vi "UHR-Fleezers Control (fpga) - 10.8a.vi"() -> ()   [LabVIEW 2014]
doc: "UHR-Fleezers Instrument Control Code (fpga)"
uses:
  <vilib>/eio/EIONode/EIONode.xnode
  <vilib>/eio/EIOMethodNode/EIOMethodNode.xnode
  <vilib>/rvi/DataTransferAndStorage/Container/XNode/niFpgaContainer.xnode
  <vilib>/Platform/TimedLoop/XDataNode/XDataNode.xnode
  <vilib>/Platform/TimedLoop/XDataNode/nitl_modes.ctl
  <vilib>/Platform/TimedLoop/XDataNode/XDNodeRunTimeDep.lvlib
  <vilib>/Platform/TimedLoop/XDataNode/wakeup.ctl
  <vilib>/Platform/TimedLoop/XDataNode/timing_clust.ctl
  <vilib>/addons/control/pid/fpga.llb/XNode/niFpgaPID.xnode
  <vilib>/rvi/eio/common/nirviEmuTemplateMethod_errors.vi
  <vilib>/rvi/interface/RandomDataEmulation/nirviRandomDataFpgaReadWriteTemplate.vi
panel:
  in  "Connector0/AO6":i16
  in  "Tab Control":T1(tab)=enum."Force FB"
  in  "Trap Pos to FIFO":bool
  in  "AI1 Sets to FIFO":T2={"Set 1"=TRUE, "Set 2"=TRUE, "Set 3"=FALSE}
  in  "N of AI1 Int Acq Sets":i16=2 min=1 max=3 step=1
  out "AI Late Counter":u16
  in  "ai count":u32=400
  out "AI late?":bool
  in  "+ phase":bool
  in  "Phase count adjustment":i16
  out "Relative phase":i16
  in  "AI to FIFO":bool
  out "BD1 Frequency Out 1":u64
  out "BD1 Frequency Out 2":u64
  out "Trap Pos FIFO Timeout":u16
  out "Trap AI FIFO Timeout":u16
  in  "Trap FIFO Set Timeout":i32
  in  "Tab Control 2":T3(tab)
  out "Wiggling 2":bool
  in  "Abort wiggle 2":bool
  in  "Wiggle amp 2":u64
  in  "Wiggle freq 2 (Hz)":fxp<+/-,16,16>
  in  "Wiggle trap 2":bool
  out "Wiggling 1":bool
  in  "Abort wiggle 1":bool
  in  "Wiggle trap 1":bool
  in  "Wiggle amp 1":u64
  in  "Wiggle freq 1 (Hz)":fxp<+/-,16,16>
  in  "Swap F1 and F2":bool
  in  "Freq or Amp switch first":bool=TRUE
  in  "Cont. Scan":bool
  in  "Abort scan":bool
  in  "Cycles per step":u64
  in  "Scan BD":bool
  in  "Number of scans":u16
  in  "Scan steps":u64
  in  "Scan freq.  increment":i64
  out "Scanning":bool
  in  "Start scan":bool
  in  "OSK Bd 1":bool
  in  "Reset Bd 1":bool
  in  "RD":bool
  in  "PMODE":bool
  in  "OSK Bd 2":bool
  in  "Reset Bd 2":bool
  in  "Direct RF Box \nCommunication":bool
  in  "Data BD 2":u8 format="%08b"
  in  "Data BD 1":u8 format="%08b"
  in  "Address":u8 format="%02x"
  in  "Update Data":bool
  in  "FPGA Controls\n RF Box":bool
  in  "Number Interlace Cycles":u8=2 min=1 max=3
  in  "Interlace Off Parameters":u8=1 min=1 max=3
  in  "Interlace ON/OFF":bool
  out "DIO Relative phase":i16
  in  "Phase count adjustment (DIO)":i16
  in  "+ phase (DIO)":bool
  out "DIO Late Counter":u16
  out "DIO Late?":bool
  in  "DIO count 1 (ticks)":u32=400
  in  "DIO count 2 (ticks)":u32=400
  in  "DIO count 3 (ticks)":u32=400
  out "AI2 Y Sum Set 2":i16
  out "AI2 Y Sum Set 1":i16
  in  "FB Gains Set 1":T4={"proportional gain (Kc)"=10, "integral gain (Kc*Ts/Ti)"=5, "derivative gain (Kc*Td/Ts)"=0}
  in  "FB Setpoint Set 1":i16 min=0 step=1
  in  "FB Reset Set 1":bool
  in  "FB On/Off Set 1":bool
  in  "FB Reset Set 2":bool
  in  "FB On/Off Set 2":bool
  in  "FB Setpoint Set 2":i16 min=0 step=1
  in  "FB Gains Set 2":T4={"proportional gain (Kc)"=10, "integral gain (Kc*Ts/Ti)"=5, "derivative gain (Kc*Td/Ts)"=0}
  in  "FB output range 2":cluster{"output high":i16, "output low":i16}={"output high"=3000, "output low"=0}
  in  "FB output range 1":cluster{"output high":i16, "output low":i16}={"output high"=3000, "output low"=0}
  out "Scan I":u64
  in  "Amp switch delay":u16=5
  in  "Freq switch delay":u16
  in  "BD 2 Amplitude 1":u16
  in  "BD 1 Amplitude 1":u16
  in  "BD 2 Frequency 1":u64
  in  "BD 1 Frequency 1":u64
  in  "BD 2 Amplitude 2":u16
  in  "BD 1 Amplitude 2":u16
  in  "BD 2 Frequency 2":u64
  in  "BD 1 Frequency 2":u64
  in  "BD 2 Amplitude 3":u16
  in  "BD 1 Amplitude 3":u16
  in  "BD 2 Frequency 3":u64
  in  "BD 1 Frequency 3":u64
  in  "Negate Diff?":bool
  in  "Diff FB Measurement?":bool
  in  "FB Trig Integrate":u32=1
  out "TTrig?":bool
  in  "TTrig Negate Pos":bool=TRUE
  out "Trap Pos FB Int Signal":fxp<+/-,24,9> format="%.18g"
  out "Trap Pos FB Int-Norm Signal":fxp<+/-,16,1> format="%.16g"
  in  "FPGA TTrig Thresh":i64
  in  "FPGA Trap Trig":bool
  out "Trap Pos FB Action":i64
  in  "Trap Pos. FB Offset Factor":i64
  in  "Trap Pos. FB Mult Factor":i64=2
  in  "Trap Pos. FB Range":T5={"output high"=0.999969482421875, "output low"=-1.0}
  in  "Trap Pos. FB Gains":T6={"proportional gain (Kc)"=0.0, "integral gain (Kc*Ts/Ti)"=10.0, "derivative gain (Kc*Td/Ts)"=0.0} {"proportional gain (Kc)" format="%.11g"; "integral gain (Kc*Ts/Ti)" format="%.11g"; "derivative gain (Kc*Td/Ts)" format="%.11g"}
  in  "Trap Pos. FB Reset":bool
  in  "Trap Pos FB Monitor T1 or T2":bool
  in  "AI1 X Scale":u16
  in  "Trap Pos FB Int Count":u16=100
  in  "Trap Pos FB Negate Action":bool
  out "AI1 X Set 2":fxp<+/-,16,1>
  out "AI1 X Set 1":fxp<+/-,16,1>
  in  "Trap Pos. FB SP":fxp<+/-,16,1>
  in  "Force feedback":bool
  out "TTrig Sig":i64
  out "TTrig Fin Thresh":i64
  out "Numeric":i32
  out "AO2 2":i16
  out "AO1 2":i16
  in  "1D or 2D Scan?":bool
  in  "Abort scan (MCL)":bool
  in  "MCL Scan Axis":bool
  in  "Cont. Scan (MCL)":bool
  out "Scan I (MCL)":u64
  in  "Number of scans (MCL)":u16
  out "Scanning MCL":bool
  in  "Scan steps (MCL)":u64
  in  "Cycles per step (MCL)":u64
  in  "Scan freq.  increment (MCL)":i16
  in  "Start scan (MCL)":bool
  in  "AO2":i16
  in  "AO1":i16
  out "MCL Late Counter":u16
  out "MCL Late?":bool
  in  "MCL count":u32=800
  out "MCL Relative Phase":i16
  in  "Phase count adjustment (MCL)":i16
  in  "+ phase (MCL)":bool
  in  "APD Gate Operating Mode":u8 max=2 step=1
  in  "Invert APD Gate":bool
  in  "APD Gate OFF Count":u32=100
  in  "APD Gate ON Count":u32=300
  out "APD 1 Gate Late Counter":u16
  out "APD 1 Gate Late?":bool
  out "APD 1 Gate Relative Phase":i16
  in  "Phase count adjustment (APD 1 Gate)":i16
  in  "+ phase (APD 1 Gate)":bool
  out "APD 2 Counts 0":u32
  out "APD 2 Counts 1":u32
  out "APD 1 Counts 0":u32
  out "APD 1 Counts 1":u32
  out "APD 1 out state":bool
  in  "APD 2 AO scale factor":i16=1
  in  "APD 1 AO scale factor":i16=1
  in  "APD to FIFO":bool
  in  "APD Acq Rate Count":u32=20000000
  out "APD Acq Late Counter":u16
  out "APD Acq Late?":bool
  out "APD Acq Relative Phase":i16
  in  "Phase Count Adjustment (APD Acq)":i16
  in  "+ phase (APD Acq)":bool
  in  "Phase count adjustment (APD 2 Gate)":i16
  out "APD 2 Gate Late Counter":u16
  out "APD 2 Gate Late?":bool
  out "APD 2 Gate Relative Phase":i16
  in  "+ phase (APD 2 Gate)":bool
  out "APD 2 out state":bool
  out "APD 1 Int Gate":bool
  out "APD 2 Int Gate":bool
  in  "Green Filter Flipper":bool
  out "Green FB Signals":T7
  in  "Green FB Count":u32=1200
  out "Green Late Counter":u16
  out "Green FB Late?":bool
  out "Green FB Relative Phase":i16
  in  "Phase count adjustment (Green FB)":i16=10
  in  "+ phase (Green FB)":bool
  out "Green FB Sum":i16
  in  "Green int current ON count adj":u32=150
  in  "Current Out":u16=30000
  in  "Green FB On/Off":bool
  in  "Green FB Setpoint":i16=250 min=0 step=1
  in  "Green FB Gains":T4={"proportional gain (Kc)"=10, "integral gain (Kc*Ts/Ti)"=5, "derivative gain (Kc*Td/Ts)"=0}
  in  "Green FB Reset":bool
  in  "Operating Mode 2":u8=2 max=2 step=1
  in  "Invert GI 2":bool
  in  "Green interlace OFF count 2":u32=900
  in  "Green interlace ON count 2":u32=300
  out "GI Late Counter 2":u16
  out "GI Late? 2":bool
  out "GI Relative phase 2":i16
  in  "Phase count adjustment (GI) 2":i16=20
  in  "+ phase (GI) 2":bool
  in  "Green interlace OFF count":u32=100
  out "GI Relative phase":i16
  in  "Phase count adjustment (GI)":i16
  in  "+ phase (GI)":bool
  in  "Green interlace ON count":u32=300
  out "GI Late Counter":u16
  in  "Invert GI":bool
  in  "Operating Mode":u8 max=2 step=1
  in  "RI Current Out":u16
  in  "RI operating mode 2":u8
  in  "Red operating mode":u8
  in  "Chassis2/Mod4/AO1":u16
  # "Only one of these can be on\nat a time:"
  # "Raster Scan AOD"
  # "1 (X)"
  # "2 (Y)"
  # "IR Intensity Feedback (RF BD 1)"
  # "FB Triggering Excitation Laser"
  # "AO1 (Y)"
  # "2D"
  # "1D"
  # "AO2 (X)"
  # "APD AO for aligning"
  # "Detection Loop"
  # "Green fluorescent laser digital gate interlacing loop"
  # "0 Forced ON\n1 Forced OFF\n2 Interlacing"
  # "Red fluorescent laser digital gate interlacing loop"
  # "0 Forced ON\n1 Forced OFF\n2 Interlacing"
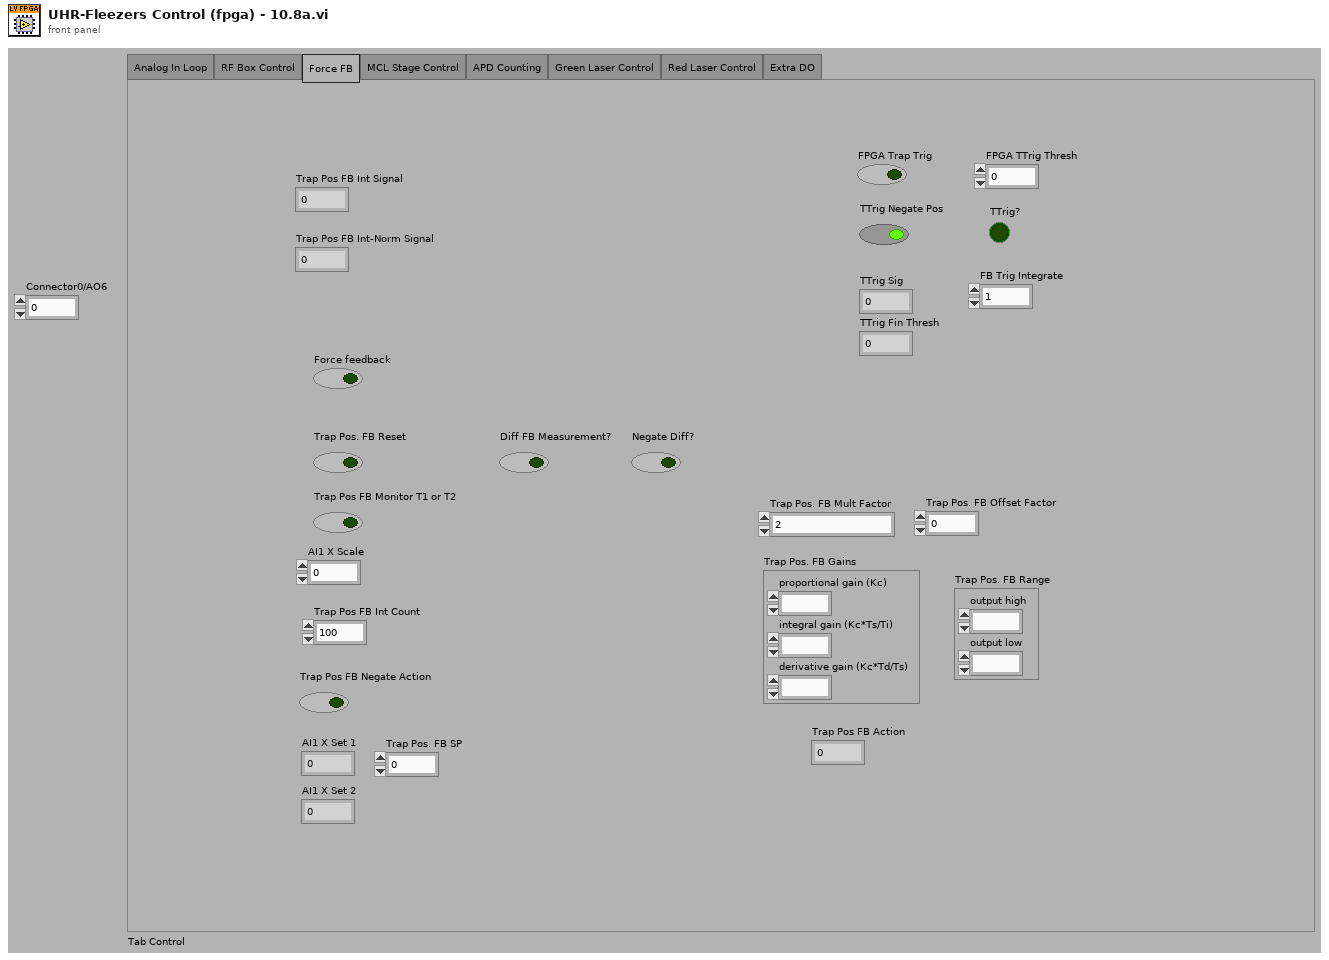
[diagram p1: front panel]
types:
  T1 = enum32{"Analog In Loop", "RF Box Control", "Force FB", "MCL Stage Control", "APD Counting", "Green Laser Control", "Red Laser Control", "Extra DO"}
  T2 = cluster{"Set 1":bool, "Set 2":bool, "Set 3":bool}
  T3 = enum32{"Controls", "Interlacing Frequency and Amplitude Values"}
  T4 = cluster{"proportional gain (Kc)":i16, "integral gain (Kc*Ts/Ti)":i16, "derivative gain (Kc*Td/Ts)":i16}
  T5 = cluster{"output high":fxp<+/-,16,1>, "output low":fxp<+/-,16,1>}
  T6 = cluster{"proportional gain (Kc)":fxp<+/-,16,8>, "integral gain (Kc*Ts/Ti)":fxp<+/-,16,8>, "derivative gain (Kc*Td/Ts)":fxp<+/-,16,8>}
  T7 = cluster{"Green FB Ch 0":i16, "Green FB Ch 1":i16, "Green FB Ch 2":i16}
  T8 = typedef "XDNodeRunTimeDep.lvlib/timing_clust.ctl" = cluster{"Expected End [f-1]":u64, "Actual End [f-1]":u64, "Finished Late? [f-1]":bool, "Expected End [i-1]":u64, "Actual End [i-1]":u64, "Finished Late? [i-1]":bool, "Expected Start [i]":u64, "Actual Start [i]":u64, "Expected Start [f]":u64, "Actual Start [f]":u64, "Source Name":string, "Structure Name":string, "Period":i64, "Deadline":i64, "Offset":i64, "Start":i64, "Priority":i32, "Timeout":i32, "Mode":T9, "Wakeup Reason":T10, "Error":errorcluster, "Source Type":string, "Secondary Source Type":string, "Global End Time":u64, "Global Start Time":u64, "Frame Duration":u64, "Iteration Duration":u64, "Assigned CPU":i32, "I/O Scan Engine Mode":u32}
  T9 = typedef "XDNodeRunTimeDep.lvlib/nitl_modes.ctl" = enum32{"No Change", "Process missed periods, maintain original phase", "Discard missed periods, maintain original phase", "Process missed periods, ignore original phase", "Discard missed periods, ignore original phase"}
  T10 = typedef "XDNodeRunTimeDep.lvlib/wakeup.ctl" = enum32{"Normal", "Aborted", "Asynchronous wakeup", "Timing source error", "Timed loop error", "Timeout"}
  T11 = cluster{"Chassis2/Mod1/AI0":void, "Chassis2/Mod1/AI1":void, "Chassis2/Mod1/AI2":void}
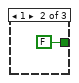
[diagram p2: hidden frame]
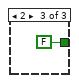
[diagram p3: hidden frame]
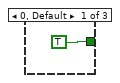
[diagram p4: hidden frame]
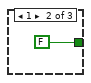
[diagram p5: hidden frame]
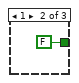
[diagram p6: hidden frame]
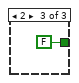
[diagram p7: hidden frame]
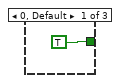
[diagram p9: hidden frame]
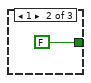
[diagram p10: hidden frame]
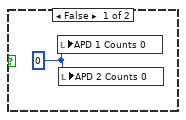
[diagram p11: hidden frame]
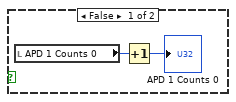
[diagram p14: hidden frame]
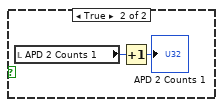
[diagram p16: hidden frame]
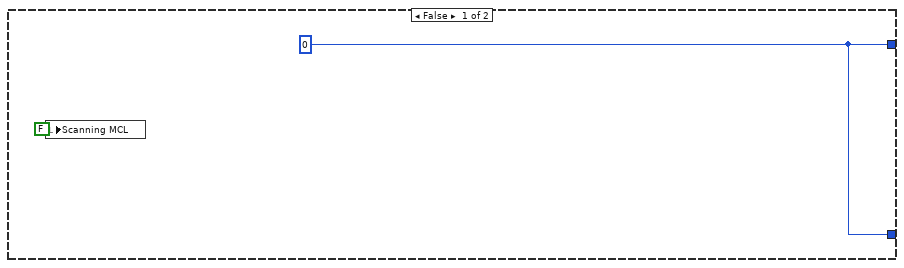
[diagram p17: hidden frame]
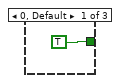
[diagram p18: hidden frame]
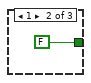
[diagram p19: hidden frame]
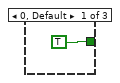
[diagram p20: hidden frame]
diagram:
  w1 = u16 0
  w4 = FALSE
  w2 = FALSE
  # "The APD Int Gate is here so the FPGA will do the integration only when the APD gate is \"ON\" (though we will leave the APD continuously ON now). This was added because the actual APD gating (via the hardware) was giving false signals. -KW"
  # "timing array current index"
  # "timing array"
  # "timing counter (phase adjusted here)"
  # "late counter"
  n1 = flat-sequence "FPGA initialization to do before running any of the loops" {
    tunnel: [u32 0 ("DIO count 3 (ticks)")] -> w3
    tunnel: [w10] -> _
    frame #0 {
      # "Start up expansion chassis early\nto avoid delays later"
      # "This pin controls udclk on the RF boards.\nWhen initially configuring the boards, this pin needs to be\nconfigured as a high impedance input.  Later it will be switched\nto an output."
      # "Initial setting of DIO data and \naddress to low (before reset).  \nThis needs to happen before the other\ncontrol method loops execute."
      n2 = xnode "FPGA I/O Node"("Chassis2/Mod4/AO0"=u16 0) -> ("Chassis2/Mod1/AI0"=w10)  [unwired: 2 in, 2 out]
      n3 = xnode "FPGA I/O Method Node"("Enable"=FALSE) -> ()  [unwired: 1 in, 1 out]
      n4 = xnode "FPGA I/O Node"("Connector1/DIO0"=FALSE, "Connector1/DIO1"=FALSE, "Connector1/DIO2"=FALSE, "Connector1/DIO3"=FALSE, "Connector1/DIO4"=FALSE, "Connector1/DIO5"=FALSE, "Connector1/DIO6"=FALSE, "Connector1/DIO7"=FALSE, "Connector1/DIO8"=FALSE, "Connector1/DIO9"=FALSE, "Connector1/DIO10"=FALSE, "Connector1/DIO11"=FALSE, "Connector1/DIO12"=FALSE, "Connector1/DIO13"=FALSE, "Connector1/DIO15"=FALSE, "Connector1/DIO20"=FALSE, "Connector1/DIO21"=FALSE, "Connector1/DIO22"=FALSE, "Connector1/DIO23"=FALSE, "Connector1/DIO24"=FALSE, "Connector1/DIO25"=FALSE, "Connector1/DIO26"=FALSE, "Connector1/DIO27"=FALSE, "Connector1/DIO14"=FALSE) -> ()  [unwired: 24 in, 24 out]
    }
  }
  n5 = local read "AO1"() -> (w8:i16)
  n6 = local read "AO2"() -> (w7:i16)
  n7 = node-c288() -> (w6:T8)  [unwired: 1 in]
  n8 = while "APD 1 Counter" {
    tunnel: w3 -> [_]
    stop <- FALSE stop-if-true
    n9 = flat-sequence {
      frame #0 {
        n10 = xnode "FPGA I/O Method Node"("FPGA I/O In"=refnum<k21> "Connector0/DIO0" ("APD 1 DO"), "Timeout"=-1) -> ()  [unwired: 2 out]
      }
      frame #1 {
        n11 = local read "APD 1 Int Gate"() -> (w41:bool)
        n12 = case shown="True" w41 {
          frame False {
          }
          frame True {
            n13 = local read "APD 1 out state"() -> (w42:bool)
            n14 = case shown="True" w42 {
              frame False {
                n15 = local read "APD 1 Counts 0"() -> (w44:u32)
                n16 = Increment(x=w44) -> (x+1=→"APD 1 Counts 0":u32)
              }
              frame True {
                n17 = local read "APD 1 Counts 1"() -> (w46:u32)
                n18 = Increment(x=w46) -> (x+1=→"APD 1 Counts 1":u32)
              }
            }
          }
        }
      }
    }
  }
  n19 = while "APD 2 Counter" {
    tunnel: w3 -> [_]
    stop <- FALSE stop-if-true
    n20 = flat-sequence {
      frame #0 {
        n21 = xnode "FPGA I/O Method Node"("FPGA I/O In"=refnum<k21> "Connector0/DIO1" ("APD 2 DO"), "Timeout"=-1) -> ()  [unwired: 2 out]
      }
      frame #1 {
        n22 = local read "APD 2 Int Gate"() -> (w50:bool)
        n23 = case shown="True" w50 {
          frame False {
          }
          frame True {
            n24 = local read "APD 2 out state"() -> (w51:bool)
            n25 = case shown="False" w51 {
              frame False {
                n26 = local read "APD 2 Counts 0"() -> (w53:u32)
                n27 = Increment(x=w53) -> (x+1=→"APD 2 Counts 0":u32)
              }
              frame True {
                n28 = local read "APD 2 Counts 1"() -> (w55:u32)
                n29 = Increment(x=w55) -> (x+1=→"APD 2 Counts 1":u32)
              }
            }
          }
        }
      }
    }
  }
  n30 = while "APD 2 Gating" {
    shift-right: [w59] -> _
    shift-left: w3 -> [w64]
    shift-right: [w58] -> _
    shift-left: w4 -> [w56]
    stop <- FALSE stop-if-true
    n31 = flat-sequence {
      tunnel: w64 -> [w67]
      tunnel: [w68] -> w62
      tunnel: [w67] -> w60
      tunnel: [w66] -> w57
      tunnel: w56 -> [w66]
      tunnel: [w71] -> w63
      tunnel: w62 -> [w71]
      tunnel: [w70] -> w61
      tunnel: w60 -> [w70]
      tunnel: w57 -> [w69]
      tunnel: [w89] -> w59
      tunnel: w63 -> [w100]
      tunnel: w61 -> [w98]
      tunnel: [w93] -> w58
      frame #0 {
        n32 = call "Loop Timer8"("Count(Ticks)"=w67) -> ("Tick Count(Ticks)"=w68:u32)
      }
      frame #1 {
        # "(need 4 channels/APD)"
        n33 = xnode "FPGA I/O Node"("Connector0/DIO8"=w69, "Connector0/DIO9"=w69, "Connector0/DIO10"=w69, "Connector0/DIO11"=w69) -> ()  [unwired: 4 in, 4 out]
        "APD 2 Int Gate" <- w69
      }
      frame #2 {
        n34 = local read "APD Gate ON Count"() -> (w82:u32)
        n35 = local read "APD Gate OFF Count"() -> (w81:u32)
        n36 = feedback #1(TRUE) -> (w95:bool)
        n37 = feedback-in #2(w100) -> ()
        n38 = feedback #2(w100) -> (w83:u32)
        n39 = Not(x=w95) -> (.not. x?=w92:bool)
        n40 = feedback-in #1(w92) -> ()
        n41 = Subtract(x=w100, y=w83) -> (x-y=w99:u32)
        n42 = Select(t=w82, s=w92, f=w81) -> (s? t:f=w97:u32)
        n43 = Subtract(x=w99, y=w98) -> (x-y=w74:u32)
        n44 = Subtract(x=w97, y=w74) -> (x-y=w88:u32)
        n45 = Number To Boolean Array(number=w74) -> (Boolean array=w73:bool[])
        n46 = Or Array Elements(Boolean array=w73) -> (logical OR=w72:bool)
        "APD 2 Gate Late?" <- w72
        n47 = Boolean To (0,1)(Boolean="+ phase (APD 2 Gate)") -> (0, 1=w86:i16)
        n48 = Multiply(x=w86, y="Phase count adjustment (APD 2 Gate)") -> (x*y=w84:i16)
        n49 = Boolean To (0,1)(Boolean=w72) -> (0, 1=w79:i16)
        n50 = Add(x=w88, y=w84) -> (x+y=w89:u32)
        n51 = To Unsigned Word Integer(number=w79) -> (unsigned 16bit integer=w76:u16)
        n52 = feedback #3(i16 0) -> (w91:i16)
        n53 = Subtract(x=w91, y=w84) -> (x-y=w90:i16)
        "APD 2 Gate Relative Phase" <- w90
        n54 = feedback-in #3(w90) -> ()
        n55 = feedback #4(u16 0) -> (w77:u16)
        n56 = Add(x=w76, y=w77) -> (x+y=w75:u16)
        "APD 2 Gate Late Counter" <- w75
        n57 = feedback-in #4(w75) -> ()
        n58 = local read "APD Gate Operating Mode"() -> (w80:u8)
        n59 = case shown="2" w80 {
          tunnel: [TRUE FALSE w106] -> w93
          tunnel: w95 -> [_ _ w104]
          frame 0, Default {
          }
          frame 1 {
          }
          frame 2 {
            n60 = local read "Invert APD Gate"() -> (w103:bool)
            n61 = Not(x=w104) -> (.not. x?=w105:bool)
            n62 = Select(t=w105, s=w103, f=w104) -> (s? t:f=w106:bool)
          }
        }
      }
    }
  }
  n63 = while "APD 1 Gating" {
    shift-right: [w110] -> _
    shift-left: w3 -> [w115]
    shift-right: [w109] -> _
    shift-left: w4 -> [w107]
    stop <- FALSE stop-if-true
    n64 = flat-sequence {
      tunnel: w115 -> [w118]
      tunnel: [w119] -> w113
      tunnel: [w118] -> w111
      tunnel: [w117] -> w108
      tunnel: w107 -> [w117]
      tunnel: [w122] -> w114
      tunnel: w113 -> [w122]
      tunnel: [w121] -> w112
      tunnel: w111 -> [w121]
      tunnel: w108 -> [w120]
      tunnel: [w136] -> w110
      tunnel: w114 -> [w151]
      tunnel: w112 -> [w148]
      tunnel: [w140] -> w109
      frame #0 {
        n65 = call "Loop Timer7"("Count(Ticks)"=w118) -> ("Tick Count(Ticks)"=w119:u32)
      }
      frame #1 {
        # "(need 4 channels/APD)"
        n66 = xnode "FPGA I/O Node"("Connector0/DIO4"=w120, "Connector0/DIO5"=w120, "Connector0/DIO6"=w120, "Connector0/DIO7"=w120) -> ()  [unwired: 4 in, 4 out]
        "APD 1 Int Gate" <- w120
      }
      frame #2 {
        n67 = feedback #5(TRUE) -> (w143:bool)
        n68 = feedback-in #6(w151) -> ()
        n69 = feedback #6(w151) -> (w150:u32)
        n70 = Not(x=w143) -> (.not. x?=w139:bool)
        n71 = feedback-in #5(w139) -> ()
        n72 = Subtract(x=w151, y=w150) -> (x-y=w149:u32)
        n73 = Select(t="APD Gate ON Count", s=w139, f="APD Gate OFF Count") -> (s? t:f=w145:u32)
        n74 = Subtract(x=w149, y=w148) -> (x-y=w124:u32)
        n75 = Subtract(x=w145, y=w124) -> (x-y=w135:u32)
        n76 = Number To Boolean Array(number=w124) -> (Boolean array=w125:bool[])
        n77 = Or Array Elements(Boolean array=w125) -> (logical OR=w123:bool)
        "APD 1 Gate Late?" <- w123
        n78 = Boolean To (0,1)(Boolean="+ phase (APD 1 Gate)") -> (0, 1=w133:i16)
        n79 = Boolean To (0,1)(Boolean=w123) -> (0, 1=w130:i16)
        n80 = Multiply(x=w133, y="Phase count adjustment (APD 1 Gate)") -> (x*y=w131:i16)
        n81 = To Unsigned Word Integer(number=w130) -> (unsigned 16bit integer=w127:u16)
        n82 = Add(x=w135, y=w131) -> (x+y=w136:u32)
        n83 = feedback #7(i16 0) -> (w138:i16)
        n84 = Subtract(x=w138, y=w131) -> (x-y=w137:i16)
        "APD 1 Gate Relative Phase" <- w137
        n85 = feedback-in #7(w137) -> ()
        n86 = feedback #8(u16 0) -> (w128:u16)
        n87 = Add(x=w127, y=w128) -> (x+y=w126:u16)
        "APD 1 Gate Late Counter" <- w126
        n88 = feedback-in #8(w126) -> ()
        n89 = case shown="2" "APD Gate Operating Mode" {
          tunnel: [TRUE FALSE w157] -> w140
          tunnel: w143 -> [_ _ w154]
          frame 0, Default {
          }
          frame 1 {
          }
          frame 2 {
            n90 = Not(x=w154) -> (.not. x?=w156:bool)
            n91 = Select(t=w156, s="Invert APD Gate", f=w154) -> (s? t:f=w157:bool)
          }
        }
      }
    }
  }
  n92 = timed-loop "RF box board DIO control: control bits" {
    timing: w6 -> [_]
    timing-out: [_] -> w5
    tunnel: [w158] -> _
    tunnel: w3 -> [w158]
    stop <- FALSE stop-if-true
    n93 = xnode "FPGA I/O Node"("Connector1/DIO16"="RD", "Connector1/DIO17"="PMODE", "Connector1/DIO18"="OSK Bd 1", "Connector1/DIO19"="Reset Bd 1", "Connector1/DIO28"="OSK Bd 2", "Connector1/DIO29"="Reset Bd 2") -> ()  [unwired: 6 in, 6 out]
  }
  n94 = while "Green fluorescent laser interlacing (DO to IA 532 nm AOM ME amp)." {
    shift-right: [w171] -> _
    shift-left: w3 -> [w176]
    shift-right: [w170] -> _
    shift-left: w2 -> [w168]
    stop <- FALSE stop-if-true
    n95 = flat-sequence {
      tunnel: w176 -> [w179]
      tunnel: [w180] -> w174
      tunnel: [w179] -> w172
      tunnel: [w178] -> w169
      tunnel: w168 -> [w178]
      tunnel: [w183] -> w175
      tunnel: w174 -> [w183]
      tunnel: [w182] -> w173
      tunnel: w172 -> [w182]
      tunnel: w169 -> [w181]
      tunnel: [w192] -> w171
      tunnel: w175 -> [w212]
      tunnel: w173 -> [w209]
      tunnel: [w201] -> w170
      frame #0 {
        n96 = call "Loop Timer4"("Count(Ticks)"=w179) -> ("Tick Count(Ticks)"=w180:u32)
      }
      frame #1 {
        n97 = xnode "FPGA I/O Node"("Connector1/DIO37"=w181, "Connector1/DIO38"=w181, "Connector1/DIO39"=w181) -> ()  [unwired: 3 in, 3 out]
      }
      frame #2 {
        n98 = feedback-in #9(w212) -> ()
        n99 = feedback #9(w212) -> (w211:u32)
        n100 = Subtract(x=w212, y=w211) -> (x-y=w210:u32)
        n101 = Subtract(x=w210, y=w209) -> (x-y=w185:u32)
        n102 = Number To Boolean Array(number=w185) -> (Boolean array=w186:bool[])
        n103 = Or Array Elements(Boolean array=w186) -> (logical OR=w184:bool)
        n104 = Boolean To (0,1)(Boolean="+ phase (GI)") -> (0, 1=w197:i16)
        n105 = Multiply(x=w197, y="Phase count adjustment (GI)") -> (x*y=w194:i16)
        n106 = Boolean To (0,1)(Boolean=w184) -> (0, 1=w191:i16)
        n107 = To Unsigned Word Integer(number=w191) -> (unsigned 16bit integer=w188:u16)
        n108 = feedback #10(i16 0) -> (w195:i16)
        n109 = feedback #11(u16 0) -> (w189:u16)
        n110 = Add(x=w188, y=w189) -> (x+y=w187:u16)
        "GI Late Counter" <- w187
        n111 = feedback-in #11(w187) -> ()
        n112 = Subtract(x=w195, y=w194) -> (x-y=w193:i16)
        "GI Relative phase" <- w193
        n113 = feedback-in #10(w193) -> ()
        n114 = feedback #12(TRUE) -> (w204:bool)
        n115 = case shown="1" "Operating Mode" {
          tunnel: [TRUE FALSE w218] -> w201
          tunnel: w204 -> [_ _ w215]
          frame 0, Default {
          }
          frame 1 {
          }
          frame 2 {
            n116 = Not(x=w215) -> (.not. x?=w217:bool)
            n117 = Select(t=w217, s="Invert GI", f=w215) -> (s? t:f=w218:bool)
          }
        }
        n118 = Not(x=w204) -> (.not. x?=w200:bool)
        n119 = Select(t="Green interlace ON count", s=w200, f="Green interlace OFF count") -> (s? t:f=w206:u32)
        n120 = Subtract(x=w206, y=w185) -> (x-y=w198:u32)
        n121 = Add(x=w198, y=w194) -> (x+y=w192:u32)
        n122 = feedback-in #12(w200) -> ()
      }
    }
  }
  n123 = while "Green fluorescent laser interlacing (Current to IA 532 nm AOM ME amp)." {
    shift-right: [w225] -> _
    shift-left: w3 -> [w228]
    shift-right: [w222] -> _
    shift-left: w1 -> [w220]
    shift-right: [w219] -> _
    shift-left: w1 -> [_]
    stop <- FALSE stop-if-true
    n124 = flat-sequence {
      tunnel: w228 -> [w231]
      tunnel: [w232] -> w227
      tunnel: [w231] -> w226
      tunnel: [w230] -> w221
      tunnel: w220 -> [w230]
      tunnel: [w235] -> w224
      tunnel: w227 -> [w235]
      tunnel: [w234] -> w223
      tunnel: w226 -> [w234]
      tunnel: w221 -> [w233]
      tunnel: [w250] -> w225
      tunnel: [w267] -> w222
      tunnel: w224 -> [w280]
      tunnel: w223 -> [w277]
      tunnel: [w236] -> w219
      frame #0 {
        n125 = call "Loop Timer10"("Count(Ticks)"=w231) -> ("Tick Count(Ticks)"=w232:u32)
      }
      frame #1 {
        n126 = xnode "FPGA I/O Node"("Chassis2/Mod4/AO0"=w233) -> ()  [unwired: 1 in, 1 out]
      }
      frame #2 {
        n127 = feedback #13(TRUE) -> (w272:bool)
        n128 = Subtract(x="Green interlace OFF count 2", y="Green int current ON count adj") -> (x-y=w259:u32)
        n129 = Not(x=w272) -> (.not. x?=w269:bool)
        n130 = feedback-in #13(w269) -> ()
        n131 = feedback-in #14(w280) -> ()
        n132 = feedback #14(w280) -> (w279:u32)
        n133 = Add(x="Green int current ON count adj", y="Green interlace ON count 2") -> (x+y=w260:u32)
        n134 = Subtract(x=w280, y=w279) -> (x-y=w278:u32)
        n135 = Select(t=w260, s=w269, f=w259) -> (s? t:f=w274:u32)
        n136 = Subtract(x=w278, y=w277) -> (x-y=w243:u32)
        n137 = case shown="0, Default" "RI operating mode 2" {
          tunnel: [TRUE FALSE FALSE] -> w240
          frame 0, Default {
          }
          frame 1 {
          }
          frame 2 {
          }
        }
        n138 = case shown="2" "Operating Mode 2" {
          tunnel: [TRUE FALSE w300] -> w261
          tunnel: w272 -> [_ _ w297]
          frame 0, Default {
          }
          frame 1 {
          }
          frame 2 {
            n139 = Not(x=w297) -> (.not. x?=w299:bool)
            n140 = Select(t=w299, s="Invert GI 2", f=w297) -> (s? t:f=w300:bool)
          }
        }
        n141 = Subtract(x=w274, y=w243) -> (x-y=w254:u32)
        n142 = Number To Boolean Array(number=w243) -> (Boolean array=w244:bool[])
        n143 = Boolean To (0,1)(Boolean="+ phase (GI) 2") -> (0, 1=w256:i16)
        n144 = Or Array Elements(Boolean array=w244) -> (logical OR=w242:bool)
        "GI Late? 2" <- w242
        n145 = Boolean To (0,1)(Boolean=w242) -> (0, 1=w249:i16)
        n146 = Multiply(x=w256, y="Phase count adjustment (GI) 2") -> (x*y=w252:i16)
        n147 = To Unsigned Word Integer(number=w249) -> (unsigned 16bit integer=w245:u16)
        n148 = Add(x=w254, y=w252) -> (x+y=w250:u32)
        n149 = feedback #15(u16 0) -> (w247:u16)
        n150 = Add(x=w245, y=w247) -> (x+y=w246:u16)
        "GI Late Counter 2" <- w246
        n151 = feedback-in #15(w246) -> ()
        n152 = feedback #16(i16 0) -> (w253:i16)
        n153 = Subtract(x=w253, y=w252) -> (x-y=w251:i16)
        "GI Relative phase 2" <- w251
        n154 = feedback-in #16(w251) -> ()
        n155 = And(x=w261, y="Green FB On/Off") -> (x .and. y?=w262:bool)
        n156 = case shown="True" w262 {
          tunnel: "Current Out" -> [w284 _]
          tunnel: [w284 w289] -> w266
          frame False {
          }
          frame True {
            n157 = local read "Green FB Sum"() -> (w285:i16)
            n158 = call "Slower PID.vi"("process variable"=w285, "reset?"="Green FB Reset", "setpoint"="Green FB Setpoint", "PID gains (x 2^8)"="Green FB Gains", "output range"=cluster{"output high":i16, "output low":i16} {"output high"=32767, "output low"=-32768} ("Green FB output range")) -> ("output"=w293:i16)  [unwired: 10 out]
            n159 = To Long Integer(number=w293) -> (32bit integer=w286:i32)
            n160 = Add(x=w286, y=32768) -> (x+y=w288:i32)
            n161 = To Unsigned Word Integer(number=w288) -> (unsigned 16bit integer=w289:u16)
          }
        }
        n162 = Boolean To (0,1)(Boolean=w240) -> (0, 1=w239:i16)
        n163 = Boolean To (0,1)(Boolean=w261) -> (0, 1=w268:i16)
        n164 = To Unsigned Word Integer(number=w268) -> (unsigned 16bit integer=w265:u16)
        n165 = To Unsigned Word Integer(number=w239) -> (unsigned 16bit integer=w238:u16)
        n166 = Multiply(x=w265, y=w266) -> (x*y=w267:u16)
        n167 = Multiply(x=w238, y="RI Current Out") -> (x*y=w236:u16)
      }
    }
  }
  n168 = while "Green excitation laser feedback measurement" {
    shift-right: [w301] -> _
    shift-left: w3 -> [w306]
    stop <- FALSE stop-if-true
    n169 = flat-sequence {
      tunnel: w306 -> [w308]
      tunnel: [w309] -> w304
      tunnel: [w308] -> w302
      tunnel: [w316] -> w305
      tunnel: w304 -> [w316]
      tunnel: [w315] -> w303
      tunnel: w302 -> [w315]
      tunnel: [w328] -> w301
      tunnel: w305 -> [w339]
      tunnel: w303 -> [w336]
      frame #0 {
        n170 = call "Loop Timer9"("Count(Ticks)"=w308) -> ("Tick Count(Ticks)"=w309:u32)
      }
      frame #1 {
        n171 = xnode "FPGA I/O Node"("Connector1/DIO35"=TRUE) -> ("Chassis2/Mod1/AI0"=w314, "Chassis2/Mod1/AI1"=w313, "Chassis2/Mod1/AI2"=w310)  [unwired: 4 in, 4 out]
        "Green FB Sum" <- w310
        n172 = Bundle("Chassis2/Mod1/AI0"=w314, "Chassis2/Mod1/AI1"=w313, "Chassis2/Mod1/AI2"=w310) -> (→"Green FB Signals":T11)  [unwired: 1 out]
      }
      frame #2 {
        n173 = feedback-in #17(w339) -> ()
        n174 = feedback #17(w339) -> (w338:u32)
        n175 = Subtract(x=w339, y=w338) -> (x-y=w337:u32)
        n176 = xnode "FPGA I/O Node"("Connector1/DIO35"=FALSE) -> ()  [unwired: 1 in, 1 out]
        n177 = Subtract(x=w337, y=w336) -> (x-y=w318:u32)
        n178 = Subtract(x="Green FB Count", y=w318) -> (x-y=w332:u32)
        n179 = Number To Boolean Array(number=w318) -> (Boolean array=w319:bool[])
        n180 = Or Array Elements(Boolean array=w319) -> (logical OR=w317:bool)
        "Green FB Late?" <- w317
        n181 = Boolean To (0,1)(Boolean="+ phase (Green FB)") -> (0, 1=w330:i16)
        n182 = Boolean To (0,1)(Boolean=w317) -> (0, 1=w324:i16)
        n183 = Multiply(x=w330, y="Phase count adjustment (Green FB)") -> (x*y=w325:i16)
        n184 = Add(x=w332, y=w325) -> (x+y=w328:u32)
        n185 = To Unsigned Word Integer(number=w324) -> (unsigned 16bit integer=w321:u16)
        n186 = feedback #18(i16 0) -> (w327:i16)
        n187 = Subtract(x=w327, y=w325) -> (x-y=w326:i16)
        "Green FB Relative Phase" <- w326
        n188 = feedback-in #18(w326) -> ()
        n189 = feedback #19(u16 0) -> (w322:u16)
        n190 = Add(x=w321, y=w322) -> (x+y=w320:u16)
        "Green Late Counter" <- w320
        n191 = feedback-in #19(w320) -> ()
      }
    }
  }
  n192 = while "Control Additional IO (Green laser flip mount)" {
    stop <- FALSE stop-if-true
    n193 = xnode "FPGA I/O Node"("Connector0/DIO3"="Green Filter Flipper", "Chassis2/Mod4/AO1"="Chassis2/Mod4/AO1", "Connector0/AO6"="Connector0/AO6") -> ()  [unwired: 3 in, 3 out]
    n194 = call "Loop Timer2"("Count(Ticks)"=u32 40000 ("Extra DO Counts")) -> ()  [unwired: 1 out]
  }
  n195 = while "DAQ AI set 1" {
    shift-right: [w345] -> _
    shift-left: w3 -> [w350]
    stop <- FALSE stop-if-true
    n196 = flat-sequence {
      tunnel: w350 -> [w360]
      tunnel: [w361] -> w348
      tunnel: [w360] -> w347
      tunnel: [w371] -> w358
      tunnel: [w370] -> w357
      tunnel: [w369] -> w356
      tunnel: [w368] -> w355
      tunnel: [w367] -> w354
      tunnel: [w366] -> w353
      tunnel: [w365] -> w352
      tunnel: [w364] -> w351
      tunnel: [w363] -> w349
      tunnel: w348 -> [w363]
      tunnel: w347 -> [w362]
      tunnel: [w362] -> w346
      tunnel: [w400] -> w345
      tunnel: w358 -> [w428]
      tunnel: w357 -> [w392]
      tunnel: w356 -> [w393]
      tunnel: w355 -> [w427]
      tunnel: w354 -> [w416]
      tunnel: w353 -> [w415]
      tunnel: w352 -> [w414]
      tunnel: w351 -> [w413]
      tunnel: w349 -> [w410]
      tunnel: w346 -> [w407]
      frame #0 {
        n197 = call "Loop Timer3"("Count(Ticks)"=w360) -> ("Tick Count(Ticks)"=w361:u32)
      }
      frame #1 {
        n198 = xnode "FPGA I/O Node"("Connector1/DIO31"=TRUE ("Connector1/DIO33")) -> ("Connector0/AI0"=w371, "Connector0/AI1"=w370, "Connector0/AI2"=w369, "Connector0/AI3"=w368, "Connector0/AI4"=w367, "Connector0/AI5"=w366, "Connector0/AI6"=w365, "Connector0/AI7"=w364)  [unwired: 9 in, 9 out]
      }
      frame #2 {
        w396 = FALSE ("AI to FIFO")
        # "Adjust phase after data acquired if button pressed"
        n199 = feedback #20(i16 1) -> (w420:i16)
        n200 = Increment(x=w420) -> (x+1=w426:i16)
        n201 = Scale By Power Of 2(n="AI1 X Scale", x=w392) -> (x*2^n=w390:dbl)
        n202 = Greater?(x=w426, y="N of AI1 Int Acq Sets") -> (0:w423:bool)
        n203 = Select(t=i16 1, s=w423, f=w426) -> (s? t:f=w425:i16)
        n204 = feedback-in #20(w425) -> ()
        n205 = Divide(x=w390, y=w393) -> (x/y=w389:fxp<+/-,16,1>)
        n206 = feedback #21(w396) -> (w394:bool)
        n207 = feedback #22(w396) -> (w412:bool)
        n208 = case shown="1, Default" w420 {
          tunnel: w393 -> [w450 w458 _]
          tunnel: "AI1 Sets to FIFO" -> [w454 w462 w468]
          tunnel: [w453 w461 w467] -> w417
          tunnel: ["AI to FIFO" w460 w466] -> w411
          tunnel: w412 -> [_ w460 w466]
          tunnel: ["Trap Pos to FIFO" w459 w465] -> w395
          tunnel: w394 -> [_ w459 w465]
          tunnel: w389 -> [w449 w457 _]
          tunnel: [w448 w455 FALSE] -> w376
          tunnel: [w447 w456 u64 0 ("BD1 Frequency Out 2")] -> w375
          frame 1, Default {
            n209 = Unbundle By Name(w454) -> ("Set 1"=w453:bool)
            n210 = local read "BD1 Frequency Out 1"() -> (w447:u64)
            n211 = Compound Arithmetic op=AND("Trap Pos to FIFO", w453, "AI to FIFO") -> (w448:bool)
            "AI2 Y Sum Set 1" <- w450
            "AI1 X Set 1" <- w449
          }
          frame 2 {
            n212 = Unbundle By Name(w462) -> ("Set 2"=w461:bool)
            n213 = local read "BD1 Frequency Out 2"() -> (w456:u64)
            n214 = Compound Arithmetic op=AND(w459, w461, w460) -> (w455:bool)
            "AI2 Y Sum Set 2" <- w458
            "AI1 X Set 2" <- w457
          }
          frame 3 {
            n215 = Unbundle By Name(w468) -> ("Set 3"=w467:bool)
          }
        }
        n216 = And(x=w417, y=w411) -> (x .and. y?=w419:bool)
        n217 = case shown="True" w419 {
          tunnel: w428 -> [_ w482]
          tunnel: w392 -> [_ w481]
          tunnel: w393 -> [_ w480]
          tunnel: w427 -> [_ w479]
          tunnel: w416 -> [_ w478]
          tunnel: w415 -> [_ w477]
          tunnel: w414 -> [_ w476]
          tunnel: w413 -> [_ w475]
          tunnel: 0 ("DMA buffer timeout") -> [_ w484]
          frame False {
          }
          frame True {
            n218 = Build Array(w482, w481, w480, w479, w478, w477, w476, w475) -> (w483:void[])
            n219 = for {
              tunnel: w483 -> [w486] mode=indexing
              tunnel: w484 -> [w487]
              tunnel: [w485] -> w473 mode=indexing
              n220 = xnode ("FIFO Write")("Element"=w486, "Timeout"=w487) -> ("Timed Out?"=w485:bool)  [unwired: 1 in, 1 out]
            }
            n221 = Or Array Elements(Boolean array=w473) -> (logical OR=w470:bool)
            n222 = Boolean To (0,1)(Boolean=w470) -> (0, 1=w472:i16)
            n223 = feedback #23(u16 0) -> (w471:u16)
            n224 = Add(x=w472, y=w471) -> (x+y=w469:u16)
            "Trap AI FIFO Timeout" <- w469
            n225 = feedback-in #23(w469) -> ()
          }
        }
        n226 = feedback-in #21(w395) -> ()
        n227 = feedback-in #22(w411) -> ()
        n228 = case shown="True" w376 {
          tunnel: w375 -> [_ w434]
          tunnel: [u8 0 w431] -> w374
          frame False {
          }
          frame True {
            n229 = Split Number(x=w434) -> (hi(x)=w435:u32, lo(x)=w436:u32)
            n230 = Split Number(x=w435) -> (lo(x)=w437:u16)  [unwired: 1 out]
            n231 = Split Number(x=w436) -> (hi(x)=w438:u16, lo(x)=w439:u16)
            n232 = Build Array "BD 1 nu Stack"(w437, w438, w439) -> (w433:u16[])
            n233 = for {
              tunnel: w433 -> [w446] mode=indexing
              shift-right: [w442] -> w431
              shift-left: u8 0 -> [w443]
              n234 = xnode ("FIFO Method Node")("Element"=w446, "Timeout"="Trap FIFO Set Timeout") -> ("Timed Out?"=w445:bool)  [unwired: 1 in, 1 out]
              n235 = Boolean To (0,1)(Boolean=w445) -> (0, 1=w444:i16)
              n236 = To Unsigned Byte Integer(number=w444) -> (unsigned 8bit integer=w441:u8)
              n237 = Add(x=w441, y=w443) -> (x+y=w442:u8)
            }
          }
        }
        n238 = To Unsigned Word Integer(number=w374) -> (unsigned 16bit integer=w373:u16)
        n239 = feedback #24(u16 0) -> (w387:u16)
        n240 = Add(x=w373, y=w387) -> (x+y=w386:u16)
        "Trap Pos FIFO Timeout" <- w386
        n241 = feedback-in #24(w386) -> ()
        n242 = feedback-in #25(w410) -> ()
        n243 = feedback #25(w410) -> (w409:u32)
        n244 = Subtract(x=w410, y=w409) -> (x-y=w408:u32)
        n245 = xnode "FPGA I/O Node"("Connector1/DIO31"=FALSE ("Connector1/DIO34")) -> ()  [unwired: 1 in, 1 out]
        n246 = Subtract(x=w408, y=w407) -> (x-y=w378:u32)
        n247 = Boolean To (0,1)(Boolean="+ phase") -> (0, 1=w403:i16)
        n248 = Multiply(x=w403, y="Phase count adjustment") -> (x*y=w397:i16)
        n249 = Subtract(x="ai count", y=w378) -> (x-y=w401:u32)
        n250 = Number To Boolean Array(number=w378) -> (Boolean array=w379:bool[])
        n251 = feedback #26(i16 0) -> (w399:i16)
        n252 = Add(x=w401, y=w397) -> (x+y=w400:u32)
        n253 = Subtract(x=w399, y=w397) -> (x-y=w398:i16)
        "Relative phase" <- w398
        n254 = feedback-in #26(w398) -> ()
        n255 = Or Array Elements(Boolean array=w379) -> (logical OR=w377:bool)
        "AI late?" <- w377
        n256 = Boolean To (0,1)(Boolean=w377) -> (0, 1=w384:i16)
        n257 = To Unsigned Word Integer(number=w384) -> (unsigned 16bit integer=w381:u16)
        n258 = feedback #27(u16 0) -> (w382:u16)
        n259 = Add(x=w381, y=w382) -> (x+y=w380:u16)
        "AI Late Counter" <- w380
        n260 = feedback-in #27(w380) -> ()
      }
    }
  }
  n261 = while "MCL stage control" {
    shift-right: [w503] -> _
    shift-left: w3 -> [w506]
    shift-right: [w496] -> _
    shift-left: w8 -> [w493]
    shift-right: [w495] -> _
    shift-left: w7 -> [w491]
    i -> [w490]
    stop <- FALSE stop-if-true
    n262 = flat-sequence {
      tunnel: w506 -> [w510]
      tunnel: [w511] -> w502
      tunnel: [w510] -> w500
      tunnel: [w509] -> w494
      tunnel: w493 -> [w509]
      tunnel: [w508] -> w492
      tunnel: w491 -> [w508]
      tunnel: w502 -> [w515]
      tunnel: [w515] -> w501
      tunnel: w500 -> [w514]
      tunnel: [w514] -> w499
      tunnel: w494 -> [w513]
      tunnel: w492 -> [w512]
      tunnel: [w513] -> w489
      tunnel: [w512] -> w488
      tunnel: w501 -> [w525]
      tunnel: w499 -> [w524]
      tunnel: [w525] -> w505
      tunnel: [w524] -> w504
      tunnel: [w523] -> w498
      tunnel: [w522] -> w497
      tunnel: w489 -> [w517]
      tunnel: w488 -> [w516]
      tunnel: [w597] -> w503
      tunnel: w505 -> [w604]
      tunnel: w504 -> [w601]
      tunnel: w498 -> [w599]
      tunnel: w497 -> [w598]
      tunnel: [w599] -> w496
      tunnel: [w598] -> w495
      frame #0 {
        n263 = call "Loop Timer5"("Count(Ticks)"=w510) -> ("Tick Count(Ticks)"=w511:u32)
      }
      frame #1 {
        n264 = xnode "FPGA I/O Node"("Connector0/AO1"=w513, "Connector0/AO2"=w512) -> ()  [unwired: 2 in, 2 out]
      }
      frame #2 {
        n265 = local read "Scanning MCL"() -> (w537:bool)
        n266 = Or(x=w537, y="Start scan (MCL)") -> (x .or. y?=w532:bool)
        n267 = Not(x="Abort scan (MCL)") -> (.not. x?=w530:bool)
        n268 = And(x=w530, y=w532) -> (x .and. y?=w529:bool)
        n269 = case "Raster scan" shown="True" w529 {
          tunnel: [w538 w581] -> w534
          tunnel: "Start scan (MCL)" -> [_ w566]
          tunnel: [w538 w542] -> w518
          frame False {
            w538 = i16 0
            n270 = local write "Scanning MCL"(FALSE ("scanning")) -> ()
          }
          frame True {
            w552 = i16 0
            w551 = u64 0
            # "scan incr."
            # "freq. incr. mult."
            # "count steps"
            # "count number of cycles"
            n271 = feedback #28(w551) -> (w578:u64)
            n272 = Select(t=w551, s=w566, f=w578) -> (s? t:f=w580:u64)
            n273 = Increment(x=w580) -> (x+1=w577:u64)
            n274 = Greater?(x="Cycles per step (MCL)", y=w577) -> (0:w561:bool)
            n275 = Select(t=w577, s=w561, f=w551) -> (s? t:f=w576:u64)
            n276 = feedback-in #28(w576) -> ()
            n277 = feedback #29(w551) -> (w575:u64)
            n278 = Select(t=w551, s=w566, f=w575) -> (s? t:f=w570:u64)
            n279 = Increment(x=w570) -> (x+1=w574:u64)
            n280 = Add(x="Scan steps (MCL)", y="Scan steps (MCL)") -> (x+y=w573:u64)
            n281 = Select(t=w570, s=w561, f=w574) -> (s? t:f=w556:u64)
            n282 = Greater?(x=w573, y=w556) -> (0:w555:bool)
            n283 = Select(t=w556, s=w555, f=w551) -> (s? t:f=w571:u64)
            n284 = feedback-in #29(w571) -> ()
            n285 = Equal?(x="Scan steps (MCL)", y=w556) -> (x = y?=w560:bool)
            n286 = Greater?(x="Scan steps (MCL)", y=w570) -> (0:w569:bool)
            n287 = feedback #30(w552) -> (w572:i16)
            n288 = Select(t=w552, s=w566, f=w572) -> (s? t:f=w558:i16)
            n289 = Increment(x=w558) -> (x+1=w568:i16)
            n290 = Decrement(x=w558) -> (x-1=w567:i16)
            n291 = Select(t=w568, s=w569, f=w567) -> (s? t:f=w559:i16)
            n292 = Select(t=w558, s=w560, f=w559) -> (s? t:f=w557:i16)
            n293 = Select(t=w558, s=w561, f=w557) -> (s? t:f=w553:i16)
            n294 = Select(t=w553, s=w555, f=w552) -> (s? t:f=w554:i16)
            n295 = feedback-in #30(w554) -> ()
            n296 = feedback #31(w551) -> (w565:u64)
            n297 = Select(t=w551, s=w566, f=w565) -> (s? t:f=w540:u64)
            n298 = Increment(x=w540) -> (x+1=w562:u64)
            n299 = Select(t=w540, s=w555, f=w562) -> (s? t:f=w541:u64)
            n300 = Greater?(x="Number of scans (MCL)", y=w541) -> (0:w548:bool)
            n301 = Multiply(x="Scan freq.  increment (MCL)", y=w558) -> (x*y=w581:i16)
            n302 = Select(t=TRUE, s="Cont. Scan (MCL)", f=w548) -> (s? t:f=w547:bool)
            "Scanning MCL" <- w547
            n303 = Select(t=w541, s=w547, f=w551) -> (s? t:f=w563:u64)
            n304 = feedback-in #31(w563) -> ()
            n305 = Increment(x=w541) -> (x+1=→"Scan I (MCL)":u64)
            n306 = To Word Integer(number=w540) -> (16bit integer=w543:i16)
            n307 = Multiply(x=w543, y="Scan freq.  increment (MCL)") -> (x*y=w542:i16)
          }
        }
        n308 = Select(t=w518, s="1D or 2D Scan?", f=i16 0) -> (s? t:f=w519:i16)
        n309 = Select(t=w519, s="MCL Scan Axis", f=w534) -> (s? t:f=w533:i16)
        n310 = Select(t=w534, s="MCL Scan Axis", f=w519) -> (s? t:f=w535:i16)
        n311 = Add(x=w533, y="AO2") -> (x+y=w522:i16)
        n312 = Add(x="AO1", y=w535) -> (x+y=w523:i16)
        "AO1 2" <- w517
        "AO2 2" <- w516
      }
      frame #3 {
        n313 = feedback-in #32(w604) -> ()
        n314 = feedback #32(w604) -> (w603:u32)
        n315 = Boolean To (0,1)(Boolean="+ phase (MCL)") -> (0, 1=w595:i16)
        n316 = Subtract(x=w604, y=w603) -> (x-y=w602:u32)
        n317 = Multiply(x=w595, y="Phase count adjustment (MCL)") -> (x*y=w591:i16)
        n318 = Subtract(x=w602, y=w601) -> (x-y=w583:u32)
        n319 = Subtract(x="MCL count", y=w583) -> (x-y=w593:u32)
        n320 = feedback #33(i16 0) -> (w592:i16)
        n321 = Subtract(x=w592, y=w591) -> (x-y=w590:i16)
        "MCL Relative Phase" <- w590
        n322 = feedback-in #33(w590) -> ()
        n323 = Number To Boolean Array(number=w583) -> (Boolean array=w584:bool[])
        n324 = Or Array Elements(Boolean array=w584) -> (logical OR=w582:bool)
        "MCL Late?" <- w582
        n325 = Boolean To (0,1)(Boolean=w582) -> (0, 1=w589:i16)
        n326 = Add(x=w593, y=w591) -> (x+y=w597:u32)
        n327 = To Unsigned Word Integer(number=w589) -> (unsigned 16bit integer=w586:u16)
        n328 = feedback #34(u16 0) -> (w587:u16)
        n329 = Add(x=w586, y=w587) -> (x+y=w585:u16)
        "MCL Late Counter" <- w585
        n330 = feedback-in #34(w585) -> ()
      }
    }
    "Numeric" <- w490
  }
  n331 = while "RF box board direct communication loop" {
    tunnel: w3 -> [_]
    stop <- FALSE stop-if-true
    n332 = case "Whether to use direct communication method (only use one method at a time)" shown="True" "Direct RF Box \nCommunication" {
      frame False {
      }
      frame True {
        n333 = case shown="True" "Update Data" {
          frame False {
          }
          frame True {
            n334 = flat-sequence {
              frame #0 {
                n335 = First Call?() -> (First Call?: T/F=w609:bool)
                n336 = case shown="True" w609 {
                  frame False {
                  }
                  frame True {
                    # "If first time data updated, be sure to set WR high\nbefore setting data and address bits."
                    n337 = flat-sequence {
                      frame #0 {
                        n338 = xnode "FPGA I/O Node"("Connector1/DIO15"=TRUE) -> ()  [unwired: 1 in, 1 out]
                      }
                      frame #1 {
                        n339 = call "Wait"("Count(Ticks)"=u8 40 ("DO Delay 3 (Ticks)")) -> ()  [unwired: 1 out]
                      }
                    }
                  }
                }
              }
              frame #1 {
                n340 = Number To Boolean Array(number="Address") -> (Boolean array=w658:bool[])
                n341 = Number To Boolean Array(number="Data BD 1") -> (Boolean array=w659:bool[])
                n342 = Number To Boolean Array(number="Data BD 2") -> (Boolean array=w628:bool[])
                n343 = Index Array(array=w659, index=7) -> (element=w643:bool)
                n344 = Index Array(array=w659, index=6) -> (element=w642:bool)
                n345 = Index Array(array=w659, index=5) -> (element=w641:bool)
                n346 = Index Array(array=w659, index=4) -> (element=w640:bool)
                n347 = Index Array(array=w659, index=3) -> (element=w639:bool)
                n348 = Index Array(array=w659, index=2) -> (element=w638:bool)
                n349 = Index Array(array=w659, index=1) -> (element=w637:bool)
                n350 = Index Array(array=w659, index=0) -> (element=w636:bool)
                n351 = Index Array(array=w658, index=5) -> (element=w635:bool)
                n352 = Index Array(array=w658, index=4) -> (element=w634:bool)
                n353 = Index Array(array=w658, index=3) -> (element=w633:bool)
                n354 = Index Array(array=w658, index=2) -> (element=w632:bool)
                n355 = Index Array(array=w658, index=1) -> (element=w631:bool)
                n356 = Index Array(array=w658, index=0) -> (element=w630:bool)
                n357 = Index Array(array=w628, index=7) -> (element=w619:bool)
                n358 = Index Array(array=w628, index=6) -> (element=w618:bool)
                n359 = Index Array(array=w628, index=5) -> (element=w617:bool)
                n360 = Index Array(array=w628, index=4) -> (element=w616:bool)
                n361 = Index Array(array=w628, index=3) -> (element=w615:bool)
                n362 = Index Array(array=w628, index=2) -> (element=w614:bool)
                n363 = Index Array(array=w628, index=1) -> (element=w613:bool)
                n364 = Index Array(array=w628, index=0) -> (element=w612:bool)
                n365 = xnode "FPGA I/O Node"("Connector1/DIO0"=w643, "Connector1/DIO1"=w642, "Connector1/DIO2"=w641, "Connector1/DIO3"=w640, "Connector1/DIO4"=w639, "Connector1/DIO5"=w638, "Connector1/DIO6"=w637, "Connector1/DIO7"=w636, "Connector1/DIO8"=w635, "Connector1/DIO9"=w634, "Connector1/DIO10"=w633, "Connector1/DIO11"=w632, "Connector1/DIO12"=w631, "Connector1/DIO13"=w630, "Connector1/DIO20"=w619, "Connector1/DIO21"=w618, "Connector1/DIO22"=w617, "Connector1/DIO23"=w616, "Connector1/DIO24"=w615, "Connector1/DIO25"=w614, "Connector1/DIO26"=w613, "Connector1/DIO27"=w612) -> ()  [unwired: 22 in, 22 out]
              }
              frame #2 {
                # "wait and then apply write signal"
                n366 = call "Wait2"("Count(Ticks)"=u8 40 ("DO Delay 1 (Ticks)")) -> ()  [unwired: 1 out]
              }
              frame #3 {
                # "sending bit low writes data to board buffer"
                n367 = xnode "FPGA I/O Node"("Connector1/DIO15"=FALSE) -> ()  [unwired: 1 in, 1 out]
              }
              frame #4 {
                # "wait then return write signal"
                n368 = call "Wait3"("Count(Ticks)"=u8 40 ("DO Delay 2 (Ticks)")) -> ()  [unwired: 1 out]
              }
              frame #5 {
                # "sending bit high makes ready to\nwrite more data"
                n369 = xnode "FPGA I/O Node"("Connector1/DIO15"=TRUE) -> ()  [unwired: 1 in, 1 out]
              }
            }
          }
        }
      }
    }
  }
  n370 = while "Control APD data integration - stream to host" {
    shift-right: [w668] -> _
    shift-left: w3 -> [w673]
    stop <- FALSE stop-if-true
    n371 = flat-sequence {
      tunnel: w673 -> [w675]
      tunnel: [w676] -> w671
      tunnel: [w675] -> w669
      tunnel: [w684] -> w672
      tunnel: w671 -> [w684]
      tunnel: [w683] -> w670
      tunnel: w669 -> [w683]
      tunnel: [w682] -> w667
      tunnel: [w681] -> w666
      tunnel: [w718] -> w668
      tunnel: w672 -> [w730]
      tunnel: w670 -> [w727]
      tunnel: w667 -> [w711]
      tunnel: w666 -> [w710]
      frame #0 {
        n372 = call "Loop Timer6"("Count(Ticks)"=w675) -> ("Tick Count(Ticks)"=w676:u32)
      }
      frame #1 {
        n373 = flat-sequence {
          tunnel: [w686] -> w680
          tunnel: w680 -> [w688]
          tunnel: [w690] -> w679
          tunnel: [w689] -> w678
          tunnel: [w688] -> w677
          tunnel: [w696] -> w681
          tunnel: [w697] -> w682
          tunnel: w679 -> [w697]
          tunnel: w678 -> [w696]
          tunnel: w677 -> [w695]
          frame #0 {
            # "use two separate variable so each APD won't\nhave to wait to read"
            n374 = feedback #35(FALSE) -> (w685:bool)
            "APD 1 out state" <- w685
            "APD 2 out state" <- w685
            n375 = Not(x=w685) -> (.not. x?=w686:bool)
            n376 = feedback-in #35(w686) -> ()
          }
          frame #1 {
            n377 = local read "APD 1 Counts 1"() -> (w694:u32)
            n378 = local read "APD 1 Counts 0"() -> (w693:u32)
            n379 = local read "APD 2 Counts 1"() -> (w692:u32)
            n380 = local read "APD 2 Counts 0"() -> (w691:u32)
            n381 = Select(t=w694, s=w688, f=w693) -> (s? t:f=w690:u32)
            n382 = Select(t=w692, s=w688, f=w691) -> (s? t:f=w689:u32)
          }
          frame #2 {
            n383 = case shown="True" w695 {
              frame False {
                w698 = u32 0 ("APD 1 Counts 0")
                n384 = local write "APD 1 Counts 0"(w698) -> ()
                n385 = local write "APD 2 Counts 0"(w698) -> ()
              }
              frame True {
                w699 = u32 0 ("APD 1 Counts 1")
                n386 = local write "APD 1 Counts 1"(w699) -> ()
                n387 = local write "APD 2 Counts 1"(w699) -> ()
              }
            }
          }
        }
      }
      frame #2 {
        n388 = feedback-in #36(w730) -> ()
        n389 = feedback #36(w730) -> (w729:u32)
        n390 = Subtract(x=w730, y=w729) -> (x-y=w728:u32)
        n391 = Subtract(x=w728, y=w727) -> (x-y=w703:u32)
        n392 = case shown="True" "APD to FIFO" {
          tunnel: w711 -> [_ w733]
          tunnel: w710 -> [_ w731]
          frame False {
          }
          frame True {
            n393 = flat-sequence {
              tunnel: 0 ("Timeout") -> [w735]
              tunnel: w733 -> [w736]
              tunnel: [w735] -> w732
              tunnel: w732 -> [w738]
              tunnel: w731 -> [w737]
              frame #0 {
                n394 = xnode ("FIFO Write")("Element"=w736, "Timeout"=w735) -> ()  [unwired: 1 in, 2 out]
              }
              frame #1 {
                n395 = xnode ("FIFO Write")("Element"=w737, "Timeout"=w738) -> ()  [unwired: 1 in, 2 out]
              }
            }
          }
        }
        n396 = Subtract(x="APD Acq Rate Count", y=w703) -> (x-y=w719:u32)
        n397 = Number To Boolean Array(number=w703) -> (Boolean array=w704:bool[])
        n398 = Or Array Elements(Boolean array=w704) -> (logical OR=w702:bool)
        "APD Acq Late?" <- w702
        n399 = Boolean To (0,1)(Boolean=w702) -> (0, 1=w709:i16)
        n400 = To Unsigned Word Integer(number=w709) -> (unsigned 16bit integer=w706:u16)
        n401 = Boolean To (0,1)(Boolean="+ phase (APD Acq)") -> (0, 1=w715:i16)
        n402 = feedback #37(u16 0) -> (w707:u16)
        n403 = Add(x=w706, y=w707) -> (x+y=w705:u16)
        "APD Acq Late Counter" <- w705
        n404 = feedback-in #37(w705) -> ()
        n405 = Multiply(x=w715, y="Phase Count Adjustment (APD Acq)") -> (x*y=w712:i16)
        n406 = Add(x=w719, y=w712) -> (x+y=w718:u32)
        n407 = feedback #38(i16 0) -> (w717:i16)
        n408 = Subtract(x=w717, y=w712) -> (x-y=w714:i16)
        "APD Acq Relative Phase" <- w714
        n409 = feedback-in #38(w714) -> ()
        n410 = To Word Integer(number=w711) -> (16bit integer=w720:i16)
        n411 = To Word Integer(number=w710) -> (16bit integer=w721:i16)
        n412 = Multiply(x="APD 1 AO scale factor", y=w720) -> (x*y=w701:i16)
        n413 = Multiply(x="APD 2 AO scale factor", y=w721) -> (x*y=w700:i16)
        n414 = xnode "FPGA I/O Node"("Connector0/AO5"=w701, "Connector0/AO7"=w700) -> ()  [unwired: 2 in, 2 out]
      }
    }
  }
  n415 = while "RF box board DIO control: parallel communication" {
    shift-right: [w745] -> _
    shift-left: w3 -> [w744]
    shift-right: [w743] -> _
    shift-left: FALSE ("Swap F1 and F2") -> [w742]
    stop <- FALSE stop-if-true
    n416 = flat-sequence {
      tunnel: w742 -> [w749]
      tunnel: w744 -> [w747]
      tunnel: [w749] -> w741
      tunnel: [w748] -> w740
      tunnel: [w747] -> w739
      tunnel: [w755] -> w745
      tunnel: [w754] -> w743
      tunnel: w741 -> [w753]
      tunnel: w740 -> [w751]
      tunnel: w739 -> [w750]
      frame #0 {
        n417 = call "Loop Timer"("Count(Ticks)"=w747) -> ("Tick Count(Ticks)"=w748:u32)
      }
      frame #1 {
        n418 = flat-sequence {
          tunnel: ["FPGA Controls\n RF Box"] -> w752
          tunnel: w753 -> [w756]
          tunnel: [w796] -> w755
          tunnel: [w809] -> w754
          tunnel: w752 -> [w808]
          tunnel: w751 -> [w802]
          tunnel: w750 -> [w799]
          frame #0 {
            n419 = case shown="True" "FPGA Controls\n RF Box" {
              tunnel: w756 -> [_ w758]
              frame False {
              }
              frame True {
                n420 = flat-sequence {
                  tunnel: w758 -> [w764]
                  frame #0 {
                    n421 = First Call?() -> (First Call?: T/F=w759:bool)
                    n422 = case shown="True" w759 {
                      frame False {
                      }
                      frame True {
                        # "If first time data updated, be sure to set WR high and UDCLK low\nbefore setting data and address bits."
                        n423 = xnode "FPGA I/O Method Node"("Enable"=TRUE) -> ("FPGA I/O Out"=w761:refnum<k21>)  [unwired: 1 in]
                        n424 = xnode "FPGA I/O Node"("Connector1/DIO15"=TRUE) -> ()  [unwired: 1 in, 1 out]
                        n425 = xnode "FPGA I/O Node"("I/O Item"=FALSE ("Connector1/DIO30"), "FPGA I/O In"=w761) -> ()  [unwired: 1 out]
                      }
                    }
                  }
                  frame #1 {
                    n426 = case shown="True" "Freq or Amp switch first" {
                      tunnel: w764 -> [w766 w771]
                      frame False {
                        n427 = flat-sequence {
                          tunnel: w766 -> [w770]
                          frame #0 {
                            # "switch amplitude"
                            # "send udclk high"
                            n428 = xnode "FPGA I/O Node"("Connector1/DIO30"=TRUE ("Connector1/DIO15")) -> ()  [unwired: 1 in, 1 out]
                          }
                          frame #1 {
                            # "send udclk low"
                            n429 = xnode "FPGA I/O Node"("Connector1/DIO30"=FALSE ("Connector1/DIO15")) -> ()  [unwired: 1 in, 1 out]
                          }
                          frame #2 {
                            n430 = call "Wait5"("Count(Ticks)"="Freq switch delay") -> ()  [unwired: 1 out]
                          }
                          frame #3 {
                            # "switch frequency"
                            n431 = xnode "FPGA I/O Node"("Connector1/DIO36"=w770) -> ()  [unwired: 1 in, 1 out]
                          }
                        }
                      }
                      frame True {
                        n432 = flat-sequence {
                          tunnel: w771 -> [w772]
                          frame #0 {
                            # "switch frequency"
                            n433 = xnode "FPGA I/O Node"("Connector1/DIO36"=w772) -> ()  [unwired: 1 in, 1 out]
                          }
                          frame #1 {
                            n434 = call "Wait4"("Count(Ticks)"="Amp switch delay") -> ()  [unwired: 1 out]
                          }
                          frame #2 {
                            # "switch amplitude"
                            # "send udclk high"
                            n435 = xnode "FPGA I/O Node"("Connector1/DIO30"=TRUE ("Connector1/DIO15")) -> ()  [unwired: 1 in, 1 out]
                          }
                          frame #3 {
                            # "send udclk low"
                            n436 = xnode "FPGA I/O Node"("Connector1/DIO30"=FALSE ("Connector1/DIO15")) -> ()  [unwired: 1 in, 1 out]
                          }
                        }
                      }
                    }
                  }
                }
              }
            }
          }
          frame #1 {
            # "This is the prior cycle's on time"
            # "increment timing\nindex, reset to 0 if \nend of matrix"
            # "Reset to begginning (1) when number of cycles reached."
            # "timing index"
            # "build byte stacks for writing data\n(must correspond to addresses array constant)"
            # "Timing housekeeping"
            # "Adjust phase if late\n(maintains constant phase relationship between cycles)"
            n437 = feedback #39(u8 0 ("t")) -> (w805:u8)
            n438 = Increment(x=w805) -> (x+1=w849:u8)
            n439 = Increment(x="Number Interlace Cycles") -> (x+1=w844:u8)
            n440 = Equal?(x=w849, y=w844) -> (x = y?=w851:bool)
            n441 = Select(t=u8 1, s=w851, f=w849) -> (s? t:f=w804:u8)
            n442 = feedback-in #39(w804) -> ()
            n443 = Increment(x=w804) -> (x+1=w846:u8)
            n444 = Equal?(x=w846, y=w844) -> (x = y?=w847:bool)
            n445 = Select(t=u8 1, s=w847, f=w846) -> (s? t:f=w843:u8)
            n446 = Select(t=w843, s="Interlace ON/OFF", f="Interlace Off Parameters") -> (s? t:f=w827:u8)
            n447 = case shown="2" w827 {
              tunnel: [w921 w1086 "BD 1 Frequency 3"] -> w839
              tunnel: [w920 "BD 2 Frequency 2" "BD 2 Frequency 3"] -> w828
              tunnel: ["BD 2 Amplitude 1" "BD 2 Amplitude 2" "BD 2 Amplitude 3"] -> w784
              tunnel: [w910 w1096 "BD 1 Amplitude 3"] -> w787
              frame 1, Default {
                w901 = fxp<+/-,24,9> 0.0 ("AI1 X Set 2")
                w894 = u16 0
                w916 = u64 0 ("f")
                # "This signal integration happens no matter what\nso that correct setpoints can be chosen before \nturning on the FB."
                # "Trap 1"
                n448 = local read "AI1 X Set 2"() -> (w897:fxp<+/-,16,1>)
                n449 = local read "AI1 X Set 1"() -> (w898:fxp<+/-,16,1>)
                n450 = local read "Scanning"() -> (w922:bool)
                n451 = case shown="False" "Diff FB Measurement?" {
                  tunnel: w897 -> [w930 w939]
                  tunnel: w898 -> [w929 w940]
                  tunnel: [w927 w931] -> w899
                  frame False {
                    n452 = Select(t=w929, s="Trap Pos FB Monitor T1 or T2", f=w930) -> (s? t:f=w927:fxp<+/-,16,1>)
                  }
                  frame True {
                    n453 = Subtract(x=w940, y=w939) -> (x-y=w932:fxp<+/-,17,2>)
                    n454 = Not(x="Negate Diff?") -> (.not. x?=w938:bool)
                    n455 = Boolean To (0,1)(Boolean="Negate Diff?") -> (0, 1=w936:i16)
                    n456 = Boolean To (0,1)(Boolean=w938) -> (0, 1=w937:i16)
                    n457 = Negate(x=w936) -> (-x=w935:i16)
                    n458 = Add(x=w935, y=w937) -> (x+y=w933:i16)
                    n459 = Multiply(x=w933, y=w932) -> (x*y=w931:fxp<+/-,32,17>)
                  }
                }
                n460 = Or(x=w922, y="Start scan") -> (x .or. y?=w914:bool)
                n461 = Not(x="Abort scan") -> (.not. x?=w912:bool)
                n462 = And(x=w912, y=w914) -> (x .and. y?=w885:bool)
                n463 = feedback #40(w894) -> (w893:u16)
                n464 = Increment(x=w893) -> (x+1=w895:u16)
                n465 = Greater Or Equal?(x=w895, y="Trap Pos FB Int Count") -> (x >= y?=w886:bool)
                n466 = case "For raster scanning" shown="False" w885 {
                  tunnel: [w1027 w1039] -> w917
                  tunnel: "Start scan" -> [_ w1063]
                  frame False {
                    # "For wiggle-calibration: sinusoidal wave"
                    n467 = local read "Wiggling 1"() -> (w1022:bool)
                    n468 = Not(x="Abort wiggle 1") -> (.not. x?=w1025:bool)
                    n469 = Or(x="Wiggle trap 1", y=w1022) -> (x .or. y?=w1021:bool)
                    n470 = And(x=w1021, y=w1025) -> (x .and. y?=w1024:bool)
                    n471 = case shown="True" w1024 {
                      tunnel: [u64 0 w1035] -> w1027
                      frame False {
                        n472 = local write "Wiggling 1"(FALSE ("Wiggle")) -> ()
                      }
                      frame True {
                        # "Input is periods/tick, not Hz,\nso need to normalize by clock\nfrequency (40 MHz)."
                        n473 = Divide(x="Wiggle freq 1 (Hz)", y=fxp<+,17,26> 40000000.0) -> (x/y=w1032:fxp<+/-,17,-9>)
                        n474 = call "Sine Wave Generator"("frequency (periods/tick)"=w1032) -> ("sine out"=w1037:i32)  [unwired: 14 in]
                        n475 = Multiply(x=w1037, y="Wiggle amp 1") -> (x*y=w1035:u64)
                        "Wiggling 1" <- TRUE
                      }
                    }
                    n476 = local write "Scanning"(FALSE ("scanning")) -> ()
                  }
                  frame True {
                    w1047 = i64 0
                    w1046 = u64 0
                    # "scan incr."
                    # "freq. incr. mult."
                    # "count steps"
                    # "count number of cycles"
                    n477 = feedback #41(w1046) -> (w1075:u64)
                    n478 = Select(t=w1046, s=w1063, f=w1075) -> (s? t:f=w1077:u64)
                    n479 = Increment(x=w1077) -> (x+1=w1074:u64)
                    n480 = Greater?(x="Cycles per step", y=w1074) -> (0:w1056:bool)
                    n481 = Select(t=w1074, s=w1056, f=w1046) -> (s? t:f=w1073:u64)
                    n482 = feedback-in #41(w1073) -> ()
                    n483 = feedback #42(w1046) -> (w1072:u64)
                    n484 = Select(t=w1046, s=w1063, f=w1072) -> (s? t:f=w1067:u64)
                    n485 = Increment(x=w1067) -> (x+1=w1071:u64)
                    n486 = Add(x="Scan steps", y="Scan steps") -> (x+y=w1070:u64)
                    n487 = Select(t=w1067, s=w1056, f=w1071) -> (s? t:f=w1051:u64)
                    n488 = Greater?(x=w1070, y=w1051) -> (0:w1050:bool)
                    n489 = Select(t=w1051, s=w1050, f=w1046) -> (s? t:f=w1068:u64)
                    n490 = feedback-in #42(w1068) -> ()
                    n491 = Equal?(x="Scan steps", y=w1051) -> (x = y?=w1055:bool)
                    n492 = Greater?(x="Scan steps", y=w1067) -> (0:w1066:bool)
                    n493 = feedback #43(w1047) -> (w1069:i64)
                    n494 = Select(t=w1047, s=w1063, f=w1069) -> (s? t:f=w1053:i64)
                    n495 = Increment(x=w1053) -> (x+1=w1065:i64)
                    n496 = Decrement(x=w1053) -> (x-1=w1064:i64)
                    n497 = Select(t=w1065, s=w1066, f=w1064) -> (s? t:f=w1054:i64)
                    n498 = Select(t=w1053, s=w1055, f=w1054) -> (s? t:f=w1052:i64)
                    n499 = Select(t=w1053, s=w1056, f=w1052) -> (s? t:f=w1048:i64)
                    n500 = Select(t=w1048, s=w1050, f=w1047) -> (s? t:f=w1049:i64)
                    n501 = feedback-in #43(w1049) -> ()
                    n502 = feedback #44(w1046) -> (w1062:u64)
                    n503 = Select(t=w1046, s=w1063, f=w1062) -> (s? t:f=w1058:u64)
                    n504 = Increment(x=w1058) -> (x+1=w1059:u64)
                    n505 = Select(t=w1058, s=w1050, f=w1059) -> (s? t:f=w1057:u64)
                    n506 = Greater?(x="Number of scans", y=w1057) -> (0:w1043:bool)
                    n507 = Multiply(x="Scan freq.  increment", y=w1053) -> (x*y=w1039:i64)
                    n508 = Select(t=TRUE, s="Cont. Scan", f=w1043) -> (s? t:f=w1042:bool)
                    "Scanning" <- w1042
                    n509 = Select(t=w1057, s=w1042, f=w1046) -> (s? t:f=w1060:u64)
                    n510 = feedback-in #44(w1060) -> ()
                    n511 = Increment(x=w1057) -> (x+1=→"Scan I":u64)
                  }
                }
                n512 = Select(t=w894, s=w886, f=w895) -> (s? t:f=w896:u16)
                n513 = feedback-in #40(w896) -> ()
                n514 = feedback #45(w901) -> (w900:fxp<+/-,24,9>)
                n515 = Add(x=w899, y=w900) -> (x+y=w892:fxp<+/-,24,9>)
                n516 = Select(t=w901, s=w886, f=w892) -> (s? t:f=w904:fxp<+/-,24,9>)
                n517 = feedback-in #45(w904) -> ()
                n518 = Divide(x=w892, y="Trap Pos FB Int Count") -> (x/y=w887:fxp<+/-,16,1>)
                n519 = feedback #46(fxp<+/-,24,9> 0.0 ("AI1 X Set 2")) -> (w905:fxp<+/-,24,9>)
                n520 = Select(t=w892, s=w886, f=w905) -> (s? t:f=w906:fxp<+/-,24,9>)
                "Trap Pos FB Int Signal" <- w906
                n521 = feedback-in #46(w906) -> ()
                n522 = feedback #47(fxp<+/-,16,1> 0.0 ("Trap Pos FB Int-Norm Signal")) -> (w889:fxp<+/-,16,1>)
                n523 = Select(t=w887, s=w886, f=w889) -> (s? t:f=w888:fxp<+/-,16,1>)
                "Trap Pos FB Int-Norm Signal" <- w888
                n524 = feedback-in #47(w888) -> ()
                n525 = case "For position feedback" shown="True" "Force feedback" {
                  tunnel: [i64 0 w946] -> w907
                  tunnel: w887 -> [_ w943]
                  tunnel: w886 -> [_ w942]
                  frame False {
                  }
                  frame True {
                    n526 = feedback #48(i64 0) -> (w945:i64)
                    n527 = case shown="True" w942 {
                      tunnel: [w947 w954] -> w946
                      tunnel: w945 -> [w947 _]
                      tunnel: w943 -> [_ w948]
                      frame False {
                      }
                      frame True {
                        w958 = u32 0
                        n528 = xnode ("PID")("process variable"=w948, "reset?"="Trap Pos. FB Reset", "setpoint"="Trap Pos. FB SP", "PID gains"="Trap Pos. FB Gains", "output range"="Trap Pos. FB Range") -> ("output"=w970:fxp<+/-,16,1>)
                        n529 = Negate(x=w970) -> (-x=w969:fxp<+/-,17,2>)
                        n530 = Select(t=w969, s="Trap Pos FB Negate Action", f=w970) -> (s? t:f=w966:fxp<+/-,17,2>)
                        n531 = Scale By Power Of 2(n=u32 15, x=u32 1) -> (x*2^n=w963:u32)
                        n532 = Multiply(x=w966, y=w963) -> (x*y=w962:fxp<+/-,17,17>)
                        n533 = To Quad Integer(1:w962) -> (0:w974:i64)
                        "Trap Pos FB Action" <- w974
                        n534 = Multiply(x=w974, y="Trap Pos. FB Mult Factor") -> (x*y=w972:i64)
                        n535 = Add(x=w972, y="Trap Pos. FB Offset Factor") -> (x+y=w954:i64)
                        n536 = feedback #49() -> (w955:i64)  [unwired: 1 in]
                        n537 = Add(x=w954, y=w955) -> (x+y=w952:i64)
                        n538 = feedback #50(w958) -> (w960:u32)
                        n539 = Increment(x=w960) -> (x+1=w949:u32)
                        n540 = Greater Or Equal?(x=w949, y="FB Trig Integrate") -> (x >= y?=w950:bool)
                        n541 = Select(t=i64 0, s=w950, f=w952) -> (s? t:f=w956:i64)
                        n542 = feedback-in #49(w956) -> ()
                        n543 = Select(t=w958, s=w950, f=w949) -> (s? t:f=w959:u32)
                        n544 = feedback-in #50(w959) -> ()
                        n545 = And(x=w950, y="FPGA Trap Trig") -> (x .and. y?=w957:bool)
                        n546 = case "Trap FB trigger excitation laser ON" shown="True" w957 {
                          tunnel: w952 -> [_ w980]
                          tunnel: w949 -> [_ w978]
                          frame False {
                          }
                          frame True {
                            n547 = Not(x="TTrig Negate Pos") -> (.not. x?=w987:bool)
                            n548 = Boolean To (0,1)(Boolean="TTrig Negate Pos") -> (0, 1=w985:i16)
                            n549 = Boolean To (0,1)(Boolean=w987) -> (0, 1=w986:i16)
                            n550 = Negate(x=w985) -> (-x=w984:i16)
                            n551 = Add(x=w984, y=w986) -> (x+y=w983:i16)
                            n552 = Multiply(x=w983, y=w980) -> (x*y=w982:i64)
                            "TTrig Sig" <- w982
                            n553 = Multiply(x="FPGA TTrig Thresh", y=w978) -> (x*y=w979:i64)
                            "TTrig Fin Thresh" <- w979
                            n554 = Greater Or Equal?(x=w982, y=w979) -> (x >= y?=w981:bool)
                            n555 = case shown="True" w981 {
                              frame False {
                              }
                              frame True {
                                w990 = TRUE ("Green FB On/Off")
                                w992 = u8 2 ("Operating Mode")
                                n556 = local write "Operating Mode 2"(w992) -> ()
                                n557 = local write "Operating Mode"(w992) -> ()
                                n558 = local write "Green FB On/Off"(w990) -> ()
                                n559 = local write "FPGA Trap Trig"(FALSE ("FPGA Trap Trig")) -> ()
                                "TTrig?" <- w990
                              }
                            }
                          }
                        }
                      }
                    }
                    n560 = feedback-in #48(w946) -> ()
                  }
                }
                n561 = case "For intensity feedback" shown="True" "FB On/Off Set 1" {
                  tunnel: "BD 1 Amplitude 1" -> [w1078 _]
                  tunnel: [w1078 w1079] -> w910
                  frame False {
                  }
                  frame True {
                    n562 = local read "AI2 Y Sum Set 1"() -> (w1081:i16)
                    n563 = call "Slower PID.vi"("process variable"=w1081, "reset?"="FB Reset Set 1", "setpoint"="FB Setpoint Set 1", "PID gains (x 2^8)"="FB Gains Set 1", "output range"="FB output range 1") -> ("output"=w1084:i16)  [unwired: 10 out]
                    n564 = To Unsigned Word Integer(number=w1084) -> (unsigned 16bit integer=w1079:u16)
                  }
                }
                n565 = Select(t=w916, s="Scan BD", f=w917) -> (s? t:f=w915:u64)
                n566 = Select(t=w917, s="Scan BD", f=w916) -> (s? t:f=w918:u64)
                n567 = Add(x=w915, y="BD 2 Frequency 1") -> (x+y=w920:u64)
                n568 = Compound Arithmetic op=ADD("BD 1 Frequency 1", w907, w918) -> (w921:u64)
                "BD1 Frequency Out 1" <- w921
              }
              frame 2 {
                # "For wiggle calibration"
                # "Trap 2"
                n569 = local read "Wiggling 2"() -> (w1093:bool)
                n570 = Or(x="Wiggle trap 2", y=w1093) -> (x .or. y?=w1092:bool)
                n571 = Not(x="Abort wiggle 2") -> (.not. x?=w1090:bool)
                n572 = And(x=w1092, y=w1090) -> (x .and. y?=w1089:bool)
                n573 = case shown="True" "FB On/Off Set 2" {
                  tunnel: [w1109 w1110] -> w1096
                  tunnel: "BD 1 Amplitude 2" -> [w1109 _]
                  frame False {
                  }
                  frame True {
                    n574 = local read "AI2 Y Sum Set 2"() -> (w1115:i16)
                    n575 = call "Slower PID.vi"("process variable"=w1115, "reset?"="FB Reset Set 2", "setpoint"="FB Setpoint Set 2", "PID gains (x 2^8)"="FB Gains Set 2", "output range"="FB output range 2") -> ("output"=w1112:i16)  [unwired: 10 out]
                    n576 = To Unsigned Word Integer(number=w1112) -> (unsigned 16bit integer=w1110:u16)
                  }
                }
                n577 = case shown="True" w1089 {
                  tunnel: [i16 0 w1103] -> w1087
                  frame False {
                    n578 = local write "Wiggling 2"(FALSE) -> ()
                  }
                  frame True {
                    n579 = Divide(x="Wiggle freq 2 (Hz)", y=fxp<+,17,26> 40000000.0) -> (x/y=w1106:fxp<+/-,17,-9>)
                    n580 = call "Sine Wave Generator2"("frequency (periods/tick)"=w1106) -> ("sine out"=w1105:i32)  [unwired: 14 in]
                    n581 = Multiply(x=w1105, y="Wiggle amp 2") -> (x*y=w1103:u64)
                    "Wiggling 2" <- TRUE
                  }
                }
                n582 = Add(x="BD 1 Frequency 2", y=w1087) -> (x+y=w1086:u64)
                "BD1 Frequency Out 2" <- w1086
              }
              frame 3 {
                # "Fluorescence period"
              }
            }
            n583 = feedback-in #51(w802) -> ()
            n584 = feedback #51(w802) -> (w801:u32)
            n585 = Select(t=w804, s="Interlace ON/OFF", f="Interlace Off Parameters") -> (s? t:f=w842:u8)
            n586 = Subtract(x=w802, y=w801) -> (x-y=w800:u32)
            n587 = Subtract "The error"(x=w800, y=w799) -> (x-y=w777:u32)
            n588 = case shown="1, Default" w842 {
              tunnel: ["DIO count 1 (ticks)" "DIO count 2 (ticks)" "DIO count 3 (ticks)"] -> w798
              frame 1, Default {
              }
              frame 2 {
              }
              frame 3 {
              }
            }
            n589 = Number To Boolean Array(number=w777) -> (Boolean array=w778:bool[])
            n590 = Or Array Elements(Boolean array=w778) -> (logical OR=w776:bool)
            "DIO Late?" <- w776
            n591 = Boolean To (0,1)(Boolean=w776) -> (0, 1=w783:i16)
            n592 = To Unsigned Word Integer(number=w783) -> (unsigned 16bit integer=w780:u16)
            n593 = feedback #52(u16 0) -> (w781:u16)
            n594 = Add(x=w780, y=w781) -> (x+y=w779:u16)
            "DIO Late Counter" <- w779
            n595 = feedback-in #52(w779) -> ()
            n596 = Subtract(x=w798, y=w777) -> (x-y=w797:u32)
            n597 = Split Number(x=w839) -> (hi(x)=w838:u32, lo(x)=w837:u32)
            n598 = Split Number(x=w828) -> (hi(x)=w833:u32, lo(x)=w832:u32)
            n599 = Boolean To (0,1)(Boolean="+ phase (DIO)") -> (0, 1=w794:i16)
            n600 = Split Number(x=w838) -> (lo(x)=w836:u16)  [unwired: 1 out]
            n601 = Split Number(x=w837) -> (hi(x)=w835:u16, lo(x)=w834:u16)
            n602 = Split Number(x=w833) -> (lo(x)=w831:u16)  [unwired: 1 out]
            n603 = Split Number(x=w832) -> (hi(x)=w830:u16, lo(x)=w829:u16)
            n604 = Split Number(x=w787) -> (hi(x)=w789:u8, lo(x)=w788:u8)
            n605 = Split Number(x=w784) -> (hi(x)=w786:u8, lo(x)=w785:u8)
            n606 = Split Number(x=w836) -> (hi(x)=w826:u8, lo(x)=w825:u8)
            n607 = Split Number(x=w835) -> (hi(x)=w824:u8, lo(x)=w823:u8)
            n608 = Split Number(x=w831) -> (hi(x)=w819:u8, lo(x)=w818:u8)
            n609 = Split Number(x=w834) -> (hi(x)=w822:u8, lo(x)=w821:u8)
            n610 = Split Number(x=w830) -> (hi(x)=w817:u8, lo(x)=w816:u8)
            n611 = Split Number(x=w829) -> (hi(x)=w815:u8, lo(x)=w814:u8)
            n612 = Multiply(x=w794, y="Phase count adjustment (DIO)") -> (x*y=w790:i16)
            n613 = feedback #53(i16 0) -> (w792:i16)
            n614 = Subtract(x=w792, y=w790) -> (x-y=w791:i16)
            "DIO Relative phase" <- w791
            n615 = feedback-in #53(w791) -> ()
            n616 = Add(x=w797, y=w790) -> (x+y=w796:u32)
            n617 = Build Array "BD 1 A Stack"(w789, w788) -> (w811:u8[])
            n618 = Build Array "BD 2 A Stack"(w786, w785) -> (w810:u8[])
            n619 = Build Array "BD 1 nu Stack"(w826, w825, w824, w823, w822, w821) -> (w820:u8[])
            n620 = Build Array "BD 2 nu Stack"(w819, w818, w817, w816, w815, w814) -> (w813:u8[])
            n621 = case shown="2" w827 {
              tunnel: [w877 w880] -> w809
              tunnel: [u8 10 u8 4] -> w812
              tunnel: "Swap F1 and F2" -> [w878 w880]
              frame 2 {
                # "F2"
                n622 = Not(x=w878) -> (.not. x?=w877:bool)
              }
              frame 1, Default {
                # "low chooses F1"
                # "F1"
              }
            }
            n623 = case "If FPGA is controlling (toggling) RF synth" shown="True" w808 {
              tunnel: w820 -> [_ w856]
              tunnel: w813 -> [_ w855]
              tunnel: w812 -> [_ w854]
              tunnel: w811 -> [_ w853]
              tunnel: w810 -> [_ w852]
              frame False {
              }
              frame True {
                # "Write next amp.\n(wait until beginning of next loop iteration to update)"
                n624 = flat-sequence "Update the next F1 and F2 frequency value (the actual frequency won't change until FSK is switched).\nThen load the next amplitude value into buffer, but don't update it until the next cycle." {
                  tunnel: w856 -> [w859]
                  tunnel: w855 -> [w858]
                  tunnel: w854 -> [w857]
                  tunnel: w853 -> [w870]
                  tunnel: w852 -> [w869]
                  frame #0 {
                    n625 = for {
                      tunnel: w859 -> [w865] mode=indexing
                      tunnel: w858 -> [w864] mode=indexing
                      tunnel: w857 -> [w862]
                      i -> [w863]
                      # "Write next freq."
                      n626 = To Unsigned Byte Integer(number=w863) -> (unsigned 8bit integer=w860:u8)
                      n627 = Add(x=w862, y=w860) -> (x+y=w861:u8)
                      n628 = call "write to RF synth bd.vi"("Address Byte"=w861, "BD 2 Byte"=w864, "BD 1 Byte"=w865) -> ()
                    }
                  }
                  frame #1 {
                    # "send udclk high"
                    n629 = xnode "FPGA I/O Node"("Connector1/DIO30"=TRUE ("Connector1/DIO15")) -> ()  [unwired: 1 in, 1 out]
                  }
                  frame #2 {
                    n630 = xnode "FPGA I/O Node"("Connector1/DIO30"=FALSE ("Connector1/DIO15")) -> ()  [unwired: 1 in, 1 out]
                  }
                  frame #3 {
                    n631 = for {
                      tunnel: w870 -> [w876] mode=indexing
                      tunnel: w869 -> [w875] mode=indexing
                      tunnel: u8 33 -> [w873]
                      i -> [w874]
                      n632 = To Unsigned Byte Integer(number=w874) -> (unsigned 8bit integer=w871:u8)
                      n633 = Add(x=w873, y=w871) -> (x+y=w872:u8)
                      n634 = call "write to RF synth bd.vi"("Address Byte"=w872, "BD 2 Byte"=w875, "BD 1 Byte"=w876) -> ()
                    }
                  }
                }
              }
            }
          }
        }
      }
    }
  }
  n635 = node-c288(w5) -> ()
  n636 = while {
    shift-right: [w1121] -> _
    shift-left: w2 -> [w1123]
    tunnel: w3 -> [w1125]
    stop <- FALSE stop-if-true
    n637 = flat-sequence {
      tunnel: w1125 -> [_]
      tunnel: [w1126] -> w1124
      tunnel: w1123 -> [w1126]
      tunnel: w1124 -> [w1127]
      tunnel: [w1128] -> w1121
      frame #0 {
      }
      frame #1 {
        n638 = xnode "FPGA I/O Node"("Connector1/DIO32"=w1127, "Connector1/DIO33"=w1127, "Connector1/DIO34"=w1127) -> ()  [unwired: 3 in, 3 out]
      }
      frame #2 {
        n639 = case shown="0, Default" "Red operating mode" {
          tunnel: [TRUE FALSE FALSE] -> w1128
          frame 0, Default {
          }
          frame 1 {
          }
          frame 2 {
          }
        }
      }
    }
  }
